vi "CFM_DAQ_SIMULACION.vi"() -> ()   [LabVIEW 2020]
panel:
  in  "stop":bool
  out "reinicio":bool
  out "M54":bool
  out "M53":bool
  out "M52":bool
  out "M51":bool
  in  "ACTUADOR RECHAZO":bool
  out "M50":bool
  out "M49":bool
  out "M48":bool
  out "M47":bool
  out "M46":bool
  out "M45":bool
  out "M44":bool
  out "TAPA NOPESO":bool
  out "M43":bool
  out "M42":bool
  out "M41":bool
  out "M40":bool
  out "M39":bool
  out "M38":bool
  out "M37":bool
  out "M36":bool
  out "M35":bool
  out "M34":bool
  out "TARRO NOPESO":bool
  out "DEPOSITO NOPESO":bool
  out "TAPA NOCOLOR":bool
  out "TARRO NOCOLOR":bool
  out "DEPOSITO NOCOLOR":bool
  out "CILINDRO RECHAZO1":bool
  out "VASTAGO RECHAZO":bool
  out "PINZA CERRADA":bool
  in  "PINZA ABIERTA":bool
  out "CILINDRO RECHAZO":bool
  out "ESTRUCTURA RECHAZO":bool
  out "M33":bool
  out "M32":bool
  out "M31":bool
  out "M30":bool
  out "M29":bool
  out "M28":bool
  out "M27":bool
  out "M26":bool
  out "TAPA AZUL":bool
  out "M25":bool
  out "M24":bool
  out "TAPA TARRO ROJO":bool
  in  "CILINDRO MODULO6":bool
  in  "VASTAGO MODULO6":bool
  in  "MODULO6":bool
  out "M23":bool
  out "M22":bool
  out "M21":bool
  out "ANALIZANDO\nCC":bool
  out "M20":bool
  out "balanza2":bool
  out "M19":bool
  out "M18":bool
  out "M17":bool
  out "M16":bool
  out "M15":bool
  out "M14":bool
  out "M13":bool
  out "M12":bool
  out "M11":bool
  out "M10":bool
  out "M9":bool
  out "M8":bool
  out "M7":bool
  out "M6":bool
  out "M5":bool
  out "M4":bool
  out "M3":bool
  out "M2":bool
  out "M1":bool
  out "tapa neutrop":bool
  out "cilindro3 tapado":bool
  out "vastago3 tapado":bool
  out "vastago4 tapado":bool
  out "cilindro2 tapado":bool
  in  "vastago2 tapado":bool
  out "cilindro1 tapado":bool
  in  "vastago1 tapado":bool
  out "estructura tapado":bool
  out "tarro llenop":bool
  out "tarro vaciop1":bool
  out "cilindros tolva":bool
  out "perta tolva1":bool
  out "puerta tolva2":bool
  out "dep inferior":bool
  out "dep superior":bool
  out "tolva vacia":bool
  out "cuadroblanco":bool
  out "vastagoaux1":bool
  out "tarro vaciop":bool
  out "estructura1":bool
  out "CILINDRO NUEVO":bool
  out "TAPA NEUTRO":bool
  out "BALANZA1":bool
  in  "BASTAGO TAPAS":bool
  out "PUERTA TOLVA":bool
  out "CAJA LLENA":bool
  out "TARRO VACIO":bool
  in  "BPESO NO":bool
  in  "BPESO SI":bool
  in  "BNO COLOR":bool
  in  "BROJO":bool
  in  "BAZUL":bool
  in  "REINICIAR\nCONTEO":bool
  out "FINALIZADOS\nRECHAZADOS":dbl
  out "FINALIZADOS\nROJOS":dbl
  out "FINALIZADOS\nAZULES":dbl
  out "AZUL":bool
  out "ROJO":bool
  out "NO \nCOLOR":bool
  out "PESO\nNO":bool
  out "PESO\nSI":bool
  in  "RESET":bool
  in  "INICIO":bool
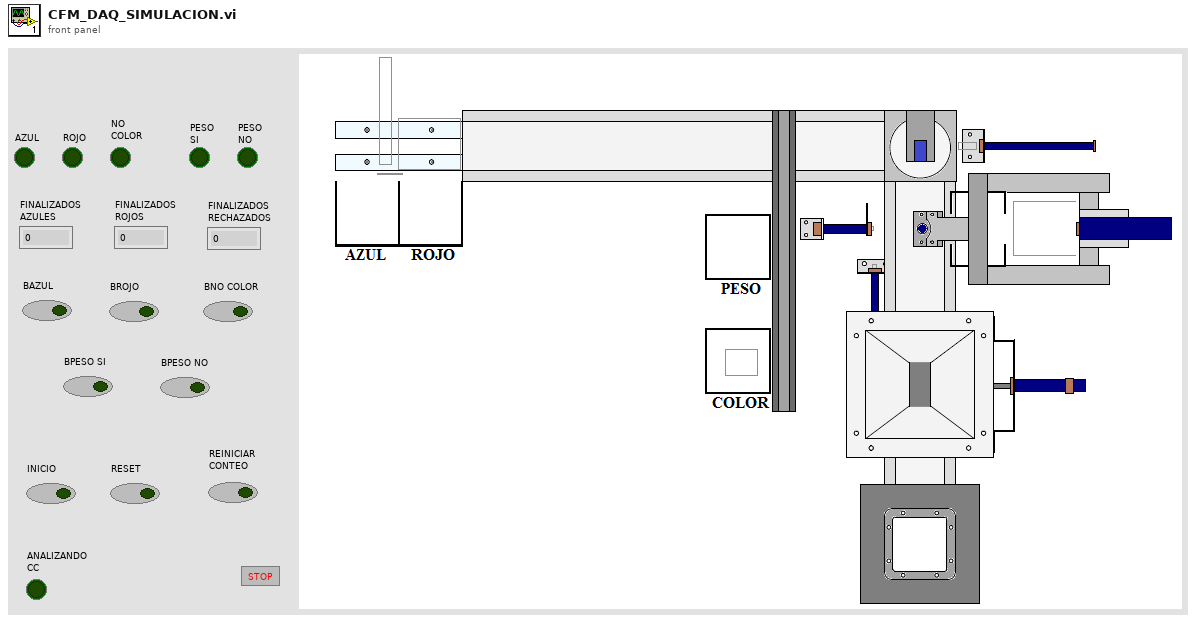
[diagram p1: front panel]
diagram:
  n1 = while {
    stop <- "stop" stop-if-true
    n2 = property on="M53" class="Bool (strict)"("Visible"=FALSE) -> ()  [unwired: 2 in, 2 out]
    n3 = property on="M54" class="Bool (strict)"("Visible"=FALSE) -> ()  [unwired: 2 in, 2 out]
    n4 = property on="M52" class="Bool (strict)"("Visible"=FALSE) -> ()  [unwired: 2 in, 2 out]
    n5 = property on="M48" class="Bool (strict)"("Visible"=FALSE) -> ()  [unwired: 2 in, 2 out]
    n6 = property on="M43" class="Bool (strict)"("Visible"=FALSE) -> ()  [unwired: 2 in, 2 out]
    n7 = property on="M47" class="Bool (strict)"("Visible"=FALSE) -> ()  [unwired: 2 in, 2 out]
    n8 = property on="M42" class="Bool (strict)"("Visible"=FALSE) -> ()  [unwired: 2 in, 2 out]
    n9 = property on="M41" class="Bool (strict)"("Visible"=FALSE) -> ()  [unwired: 2 in, 2 out]
    n10 = property on="M49" class="Bool (strict)"("Visible"=FALSE) -> ()  [unwired: 2 in, 2 out]
    n11 = property on="M40" class="Bool (strict)"("Visible"=FALSE) -> ()  [unwired: 2 in, 2 out]
    n12 = property on="M45" class="Bool (strict)"("Visible"=FALSE) -> ()  [unwired: 2 in, 2 out]
    n13 = property on="M46" class="Bool (strict)"("Visible"=FALSE) -> ()  [unwired: 2 in, 2 out]
    n14 = property on="reinicio" class="Bool (strict)"("Visible"=FALSE) -> ()  [unwired: 2 in, 2 out]
    n15 = property on="M24" class="Bool (strict)"("Visible"=FALSE) -> ()  [unwired: 2 in, 2 out]
    n16 = property on="M39" class="Bool (strict)"("Visible"=FALSE) -> ()  [unwired: 2 in, 2 out]
    n17 = property on="M44" class="Bool (strict)"("Visible"=FALSE) -> ()  [unwired: 2 in, 2 out]
    n18 = property on="M50" class="Bool (strict)"("Visible"=FALSE) -> ()  [unwired: 2 in, 2 out]
    n19 = property on="M25" class="Bool (strict)"("Visible"=FALSE) -> ()  [unwired: 2 in, 2 out]
    n20 = property on="M37" class="Bool (strict)"("Visible"=FALSE) -> ()  [unwired: 2 in, 2 out]
    n21 = property on="M38" class="Bool (strict)"("Visible"=FALSE) -> ()  [unwired: 2 in, 2 out]
    n22 = property on="M23" class="Bool (strict)"("Visible"=FALSE) -> ()  [unwired: 2 in, 2 out]
    n23 = property on="M22" class="Bool (strict)"("Visible"=FALSE) -> ()  [unwired: 2 in, 2 out]
    n24 = property on="M51" class="Bool (strict)"("Visible"=FALSE) -> ()  [unwired: 2 in, 2 out]
    n25 = property on="M36" class="Bool (strict)"("Visible"=FALSE) -> ()  [unwired: 2 in, 2 out]
    n26 = property on="M21" class="Bool (strict)"("Visible"=FALSE) -> ()  [unwired: 2 in, 2 out]
    n27 = property on="M27" class="Bool (strict)"("Visible"=FALSE) -> ()  [unwired: 2 in, 2 out]
    n28 = property on="M33" class="Bool (strict)"("Visible"=FALSE) -> ()  [unwired: 2 in, 2 out]
    n29 = property on="M2" class="Bool (strict)"("Visible"=FALSE) -> ()  [unwired: 2 in, 2 out]
    n30 = property on="M26" class="Bool (strict)"("Visible"=FALSE) -> ()  [unwired: 2 in, 2 out]
    n31 = property on="M35" class="Bool (strict)"("Visible"=FALSE) -> ()  [unwired: 2 in, 2 out]
    n32 = property on="M1" class="Bool (strict)"("Visible"=FALSE) -> ()  [unwired: 2 in, 2 out]
    n33 = property on="M32" class="Bool (strict)"("Visible"=FALSE) -> ()  [unwired: 2 in, 2 out]
    n34 = property on="M34" class="Bool (strict)"("Visible"=FALSE) -> ()  [unwired: 2 in, 2 out]
    n35 = property on="M13" class="Bool (strict)"("Visible"=FALSE) -> ()  [unwired: 2 in, 2 out]
    n36 = property on="M20" class="Bool (strict)"("Visible"=FALSE) -> ()  [unwired: 2 in, 2 out]
    n37 = property on="M29" class="Bool (strict)"("Visible"=FALSE) -> ()  [unwired: 2 in, 2 out]
    n38 = property on="M15" class="Bool (strict)"("Visible"=FALSE) -> ()  [unwired: 2 in, 2 out]
    n39 = property on="M28" class="Bool (strict)"("Visible"=FALSE) -> ()  [unwired: 2 in, 2 out]
    n40 = property on="M5" class="Bool (strict)"("Visible"=FALSE) -> ()  [unwired: 2 in, 2 out]
    n41 = property on="M3" class="Bool (strict)"("Visible"=FALSE) -> ()  [unwired: 2 in, 2 out]
    n42 = property on="M18" class="Bool (strict)"("Visible"=FALSE) -> ()  [unwired: 2 in, 2 out]
    n43 = property on="M19" class="Bool (strict)"("Visible"=FALSE) -> ()  [unwired: 2 in, 2 out]
    n44 = property on="M8" class="Bool (strict)"("Visible"=FALSE) -> ()  [unwired: 2 in, 2 out]
    n45 = property on="M7" class="Bool (strict)"("Visible"=FALSE) -> ()  [unwired: 2 in, 2 out]
    n46 = property on="M30" class="Bool (strict)"("Visible"=FALSE) -> ()  [unwired: 2 in, 2 out]
    n47 = property on="M6" class="Bool (strict)"("Visible"=FALSE) -> ()  [unwired: 2 in, 2 out]
    n48 = property on="M9" class="Bool (strict)"("Visible"=FALSE) -> ()  [unwired: 2 in, 2 out]
    n49 = property on="M17" class="Bool (strict)"("Visible"=FALSE) -> ()  [unwired: 2 in, 2 out]
    n50 = property on="M4" class="Bool (strict)"("Visible"=FALSE) -> ()  [unwired: 2 in, 2 out]
    n51 = property on="M10" class="Bool (strict)"("Visible"=FALSE) -> ()  [unwired: 2 in, 2 out]
    n52 = property on="M11" class="Bool (strict)"("Visible"=FALSE) -> ()  [unwired: 2 in, 2 out]
    n53 = property on="M14" class="Bool (strict)"("Visible"=FALSE) -> ()  [unwired: 2 in, 2 out]
    n54 = property on="M16" class="Bool (strict)"("Visible"=FALSE) -> ()  [unwired: 2 in, 2 out]
    n55 = property on="M12" class="Bool (strict)"("Visible"=FALSE) -> ()  [unwired: 2 in, 2 out]
    n56 = property on="M31" class="Bool (strict)"("Visible"=FALSE) -> ()  [unwired: 2 in, 2 out]
    n57 = property on="ACTUADOR RECHAZO" class="Bool (strict)"() -> ("Top"=w82:i32)  [unwired: 2 in, 2 out]
    n58 = property on="ACTUADOR RECHAZO" class="Bool (strict)"() -> ("Top"=w67:i32)  [unwired: 2 in, 2 out]
    n59 = property on="ACTUADOR RECHAZO" class="Bool (strict)"() -> ("Top"=w97:i32)  [unwired: 2 in, 2 out]
    n60 = property on="ACTUADOR RECHAZO" class="Bool (strict)"() -> ("Top"=w154:i32)  [unwired: 2 in, 2 out]
    n61 = local read "BNO COLOR"() -> (w121:bool)
    n62 = property on="ACTUADOR RECHAZO" class="Bool (strict)"() -> ("Top"=w139:i32)  [unwired: 2 in, 2 out]
    n63 = property on="VASTAGO MODULO6" class="Bool (strict)"() -> ("Top"=w232:i32)  [unwired: 2 in, 2 out]
    n64 = property on="VASTAGO MODULO6" class="Bool (strict)"() -> ("Top"=w195:i32)  [unwired: 2 in, 2 out]
    n65 = property on="VASTAGO MODULO6" class="Bool (strict)"() -> ("Top"=w190:i32)  [unwired: 2 in, 2 out]
    n66 = property on="VASTAGO MODULO6" class="Bool (strict)"() -> ("Top"=w237:i32)  [unwired: 2 in, 2 out]
    n67 = local read "BPESO NO"() -> (w122:bool)
    n68 = property on="TAPA TARRO ROJO" class="Bool (strict)"() -> ("Left"=w242:i32)  [unwired: 2 in, 2 out]
    n69 = local read "BPESO NO"() -> (w168:bool)
    n70 = property on="PINZA CERRADA" class="Bool (strict)"() -> ("Top"=w77:i32)  [unwired: 2 in, 2 out]
    n71 = property on="PINZA CERRADA" class="Bool (strict)"() -> ("Top"=w129:i32)  [unwired: 2 in, 2 out]
    n72 = property on="PINZA CERRADA" class="Bool (strict)"() -> ("Top"=w87:i32)  [unwired: 2 in, 2 out]
    n73 = property on="PINZA CERRADA" class="Bool (strict)"() -> ("Top"=w72:i32)  [unwired: 2 in, 2 out]
    n74 = property on="vastago4 tapado" class="Bool (strict)"() -> ("Top"=w300:i32)  [unwired: 2 in, 2 out]
    n75 = property on="TAPA NOCOLOR" class="Bool (strict)"() -> ("Left"=w159:i32)  [unwired: 2 in, 2 out]
    n76 = property on="BASTAGO TAPAS" class="Bool (strict)"() -> ("Left"=w305:i32)  [unwired: 2 in, 2 out]
    n77 = property on="PINZA CERRADA" class="Bool (strict)"() -> ("Top"=w149:i32)  [unwired: 2 in, 2 out]
    n78 = property on="PINZA CERRADA" class="Bool (strict)"() -> ("Top"=w144:i32)  [unwired: 2 in, 2 out]
    n79 = property on="vastago4 tapado" class="Bool (strict)"() -> ("Top"=w295:i32)  [unwired: 2 in, 2 out]
    n80 = property on="CILINDRO NUEVO" class="Bool (strict)"() -> ("Left"=w290:i32)  [unwired: 2 in, 2 out]
    n81 = property on="PINZA CERRADA" class="Bool (strict)"() -> ("Top"=w92:i32)  [unwired: 2 in, 2 out]
    n82 = property on="vastago3 tapado" class="Bool (strict)"() -> ("Top"=w280:i32)  [unwired: 2 in, 2 out]
    n83 = local read "BNO COLOR"() -> (w169:bool)
    n84 = property on="PINZA CERRADA" class="Bool (strict)"() -> ("Top"=w134:i32)  [unwired: 2 in, 2 out]
    n85 = property on="TAPA NOPESO" class="Bool (strict)"() -> ("Left"=w102:i32)  [unwired: 2 in, 2 out]
    n86 = property on="balanza2" class="Bool (strict)"() -> ("Left"=w109:i32)  [unwired: 2 in, 2 out]
    n87 = property on="TAPA NEUTRO" class="Bool (strict)"() -> ("Top"=w275:i32)  [unwired: 2 in, 2 out]
    n88 = property on="TAPA NEUTRO" class="Bool (strict)"() -> ("Top"=w265:i32)  [unwired: 2 in, 2 out]
    n89 = property on="PUERTA TOLVA" class="Bool (strict)"() -> ("Left"=w330:i32)  [unwired: 2 in, 2 out]
    n90 = property on="PUERTA TOLVA" class="Bool (strict)"() -> ("Left"=w325:i32)  [unwired: 2 in, 2 out]
    n91 = property on="tapa neutrop" class="Bool (strict)"() -> ("Top"=w285:i32)  [unwired: 2 in, 2 out]
    n92 = property on="TARRO VACIO" class="Bool (strict)"() -> ("Top"=w335:i32)  [unwired: 2 in, 2 out]
    n93 = property on="vastagoaux1" class="Bool (strict)"() -> ("Top"=w345:i32)  [unwired: 2 in, 2 out]
    n94 = local read "BPESO SI"() -> (w224:bool)
    n95 = property on="balanza2" class="Bool (strict)"() -> ("Left"=w119:i32)  [unwired: 2 in, 2 out]
    n96 = local read "BPESO SI"() -> (w230:bool)
    n97 = property on="puerta tolva2" class="Bool (strict)"() -> ("Left"=w320:i32)  [unwired: 2 in, 2 out]
    n98 = property on="puerta tolva2" class="Bool (strict)"() -> ("Left"=w315:i32)  [unwired: 2 in, 2 out]
    n99 = local read "BPESO NO"() -> (w124:bool)
    n100 = property on="vastagoaux1" class="Bool (strict)"() -> ("Top"=w350:i32)  [unwired: 2 in, 2 out]
    n101 = property on="vastagoaux1" class="Bool (strict)"() -> ("Top"=w340:i32)  [unwired: 2 in, 2 out]
    n102 = property on="TAPA AZUL" class="Bool (strict)"() -> ("Left"=w205:i32)  [unwired: 2 in, 2 out]
    n103 = property on="MODULO6" class="Bool (strict)"() -> ("Left"=w200:i32)  [unwired: 2 in, 2 out]
    n104 = property on="MODULO6" class="Bool (strict)"() -> ("Left"=w185:i32)  [unwired: 2 in, 2 out]
    n105 = property on="CAJA LLENA" class="Bool (strict)"() -> ("Top"=w310:i32)  [unwired: 2 in, 2 out]
    n106 = property on="BALANZA1" class="Bool (strict)"() -> ("Top"=w270:i32)  [unwired: 2 in, 2 out]
    n107 = property on="balanza2" class="Bool (strict)"() -> ("Left"=w114:i32)  [unwired: 2 in, 2 out]
    n108 = property on="balanza2" class="Bool (strict)"() -> ("Left"=w220:i32)  [unwired: 2 in, 2 out]
    n109 = local read "BROJO"() -> (w229:bool)
    n110 = local read "BAZUL"() -> (w225:bool)
    n111 = property on="balanza2" class="Bool (strict)"() -> ("Left"=w259:i32)  [unwired: 2 in, 2 out]
    n112 = property on="balanza2" class="Bool (strict)"() -> ("Left"=w164:i32)  [unwired: 2 in, 2 out]
    n113 = property on="balanza2" class="Bool (strict)"() -> ("Left"=w210:i32)  [unwired: 2 in, 2 out]
    n114 = property on="balanza2" class="Bool (strict)"() -> ("Left"=w176:i32)  [unwired: 2 in, 2 out]
    n115 = property on="balanza2" class="Bool (strict)"() -> ("Left"=w247:i32)  [unwired: 2 in, 2 out]
    n116 = property on="balanza2" class="Bool (strict)"() -> ("Left"=w215:i32)  [unwired: 2 in, 2 out]
    n117 = property on="balanza2" class="Bool (strict)"() -> ("Left"=w171:i32)  [unwired: 2 in, 2 out]
    n118 = property on="balanza2" class="Bool (strict)"() -> ("Left"=w252:i32)  [unwired: 2 in, 2 out]
    n119 = local read "reinicio"() -> (w63:bool)
    n120 = local read "INICIO"() -> (w64:bool)
    n121 = Not(x=w168) -> (.not. x?=w180:bool)
    n122 = local read "M46"() -> (w106:bool)
    n123 = And(x=w122, y=w121) -> (x .and. y?=w123:bool)
    n124 = Less?(x=w119, y=965) -> (x < y?=w120:bool)
    n125 = local read "M52"() -> (w79:bool)
    n126 = local read "M47"() -> (w104:bool)
    n127 = local read "M45"() -> (w111:bool)
    n128 = local read "M43"() -> (w131:bool)
    n129 = local read "M50"() -> (w89:bool)
    n130 = local read "M44"() -> (w116:bool)
    n131 = Greater?(x=w109, y=977) -> (0:w110:bool)
    n132 = local read "M51"() -> (w84:bool)
    n133 = local read "M54"() -> (w69:bool)
    n134 = local read "M19"() -> (w262:bool)
    n135 = local read "M25"() -> (w234:bool)
    n136 = local read "M26"() -> (w222:bool)
    n137 = local read "M36"() -> (w166:bool)
    n138 = local read "M37"() -> (w161:bool)
    n139 = local read "M53"() -> (w74:bool)
    n140 = local read "M28"() -> (w212:bool)
    n141 = local read "M48"() -> (w99:bool)
    n142 = local read "M10"() -> (w307:bool)
    n143 = local read "M14"() -> (w287:bool)
    n144 = local read "M16"() -> (w277:bool)
    n145 = local read "M20"() -> (w257:bool)
    n146 = local read "M30"() -> (w202:bool)
    n147 = local read "M31"() -> (w197:bool)
    n148 = local read "M33"() -> (w187:bool)
    n149 = local read "M39"() -> (w151:bool)
    n150 = local read "M40"() -> (w146:bool)
    n151 = local read "M23"() -> (w244:bool)
    n152 = local read "M29"() -> (w207:bool)
    n153 = local read "M34"() -> (w178:bool)
    n154 = local read "M41"() -> (w141:bool)
    n155 = local read "M12"() -> (w297:bool)
    n156 = local read "M19"() -> (w227:bool)
    n157 = local read "M32"() -> (w192:bool)
    n158 = local read "M19"() -> (w182:bool)
    n159 = local read "M38"() -> (w156:bool)
    n160 = local read "M49"() -> (w94:bool)
    n161 = local read "M11"() -> (w302:bool)
    n162 = local read "M17"() -> (w272:bool)
    n163 = local read "M18"() -> (w267:bool)
    n164 = local read "M22"() -> (w249:bool)
    n165 = local read "M24"() -> (w239:bool)
    n166 = local read "M27"() -> (w217:bool)
    n167 = local read "M35"() -> (w173:bool)
    n168 = local read "M42"() -> (w136:bool)
    n169 = local read "M19"() -> (w126:bool)
    n170 = local read "M2"() -> (w347:bool)
    n171 = local read "M15"() -> (w282:bool)
    n172 = local read "M1"() -> (w352:bool)
    n173 = local read "M21"() -> (w254:bool)
    n174 = local read "M4"() -> (w337:bool)
    n175 = local read "M13"() -> (w292:bool)
    n176 = local read "M6"() -> (w327:bool)
    n177 = local read "M8"() -> (w317:bool)
    n178 = Less?(x=w114, y=900) -> (x < y?=w115:bool)
    n179 = local read "M3"() -> (w342:bool)
    n180 = local read "M5"() -> (w332:bool)
    n181 = local read "M9"() -> (w312:bool)
    n182 = local read "M7"() -> (w322:bool)
    n183 = Equal?(x=420, y=w350) -> (x = y?=w351:bool)
    n184 = Less?(x=w102, y=737) -> (x < y?=w103:bool)
    n185 = property on="BAZUL" class="Bool (strict)"("Visible"=TRUE) -> ()  [unwired: 2 in, 2 out]
    n186 = Greater?(x=w195, y=55) -> (0:w196:bool)
    n187 = Less?(x=w129, y=317) -> (x < y?=w130:bool)
    n188 = Greater?(x=w77, y=396) -> (0:w78:bool)
    n189 = And(x=w229, y=w230) -> (x .and. y?=w261:bool)
    n190 = Less?(x=w275, y=67) -> (x < y?=w276:bool)
    n191 = And(x=w225, y=w224) -> (x .and. y?=w226:bool)
    n192 = Less?(x=w205, y=426) -> (x < y?=w206:bool)
    n193 = Greater?(x=w139, y=219) -> (0:w140:bool)
    n194 = Less?(x=w97, y=6) -> (x < y?=w98:bool)
    n195 = Less?(x=w87, y=317) -> (x < y?=w88:bool)
    n196 = property on="BROJO" class="Bool (strict)"("Visible"=TRUE) -> ()  [unwired: 2 in, 2 out]
    n197 = Less?(x=w232, y=-10) -> (x < y?=w233:bool)
    n198 = Less?(x=w159, y=737) -> (x < y?=w160:bool)
    n199 = Greater?(x=w67, y=219) -> (0:w68:bool)
    n200 = Less?(x=w305, y=911) -> (x < y?=w306:bool)
    n201 = Greater?(x=w285, y=367) -> (0:w286:bool)
    n202 = Less?(x=w215, y=900) -> (x < y?=w216:bool)
    n203 = Greater?(x=w210, y=977) -> (0:w211:bool)
    n204 = Greater?(x=w185, y=377) -> (0:w186:bool)
    n205 = Less?(x=w144, y=317) -> (x < y?=w145:bool)
    n206 = Greater?(x=w92, y=396) -> (0:w93:bool)
    n207 = Greater?(x=w340, y=383) -> (0:w341:bool)
    n208 = Less?(x=w335, y=252) -> (x < y?=w336:bool)
    n209 = Greater?(x=w300, y=258) -> (0:w301:bool)
    n210 = Less?(x=w259, y=965) -> (x < y?=w256:bool)
    n211 = Greater?(x=w237, y=38) -> (0:w238:bool)
    n212 = And(x=w169, y=w180) -> (x .and. y?=w181:bool)
    n213 = Less?(x=w72, y=317) -> (x < y?=w73:bool)
    n214 = Less?(x=w242, y=426) -> (x < y?=w243:bool)
    n215 = Less?(x=w220, y=965) -> (x < y?=w221:bool)
    n216 = Less?(x=w200, y=316) -> (x < y?=w201:bool)
    n217 = Less?(x=w190, y=10) -> (x < y?=w191:bool)
    n218 = Less?(x=w176, y=965) -> (x < y?=w177:bool)
    n219 = Less?(x=w171, y=900) -> (x < y?=w172:bool)
    n220 = Greater?(x=w164, y=977) -> (0:w165:bool)
    n221 = Less?(x=w154, y=6) -> (x < y?=w155:bool)
    n222 = Greater?(x=w134, y=396) -> (0:w135:bool)
    n223 = Or(x=w124, y=w123) -> (x .or. y?=w125:bool)
    n224 = Less?(x=w325, y=931) -> (x < y?=w326:bool)
    n225 = Less?(x=w295, y=227) -> (x < y?=w296:bool)
    n226 = Less?(x=w270, y=109) -> (x < y?=w271:bool)
    n227 = Greater?(x=w247, y=977) -> (0:w248:bool)
    n228 = Greater?(x=w149, y=396) -> (0:w150:bool)
    n229 = Greater?(x=w82, y=100) -> (0:w83:bool)
    n230 = Less?(x=w345, y=386) -> (x < y?=w346:bool)
    n231 = Less?(x=w320, y=425) -> (x < y?=w321:bool)
    n232 = Less?(x=w310, y=97) -> (x < y?=w311:bool)
    n233 = Less?(x=w265, y=16) -> (x < y?=w266:bool)
    n234 = Greater?(x=w315, y=449) -> (0:w316:bool)
    n235 = Less?(x=w290, y=870) -> (x < y?=w291:bool)
    n236 = Greater?(x=w330, y=950) -> (0:w331:bool)
    n237 = Less?(x=w280, y=207) -> (x < y?=w281:bool)
    n238 = Less?(x=w252, y=900) -> (x < y?=w253:bool)
    n239 = local read "RESET"() -> (w62:bool)
    n240 = Or(x=w64, y=w63) -> (x .or. y?=w65:bool)
    n241 = And(x=w277, y=w276) -> (x .and. y?=w278:bool)
    n242 = And(x=w161, y=w160) -> (x .and. y?=w162:bool)
    n243 = And(x=w352, y=w351) -> (x .and. y?=w353:bool)
    n244 = And(x=w287, y=w286) -> (x .and. y?=w288:bool)
    n245 = And(x=w234, y=w233) -> (x .and. y?=w235:bool)
    n246 = And(x=w146, y=w145) -> (x .and. y?=w147:bool)
    n247 = And(x=w131, y=w130) -> (x .and. y?=w132:bool)
    n248 = And(x=w111, y=w115) -> (x .and. y?=w112:bool)
    n249 = And(x=w106, y=w110) -> (x .and. y?=w107:bool)
    n250 = And(x=w79, y=w78) -> (x .and. y?=w80:bool)
    n251 = And(x=w337, y=w336) -> (x .and. y?=w338:bool)
    n252 = And(x=w227, y=w226) -> (x .and. y?=w228:bool)
    n253 = And(x=w222, y=w221) -> (x .and. y?=w223:bool)
    n254 = And(x=w178, y=w177) -> (x .and. y?=w179:bool)
    n255 = And(x=w166, y=w165) -> (x .and. y?=w167:bool)
    n256 = And(x=w116, y=w120) -> (x .and. y?=w117:bool)
    n257 = And(x=w347, y=w346) -> (x .and. y?=w348:bool)
    n258 = And(x=w327, y=w326) -> (x .and. y?=w328:bool)
    n259 = And(x=w272, y=w271) -> (x .and. y?=w273:bool)
    n260 = And(x=w244, y=w243) -> (x .and. y?=w245:bool)
    n261 = And(x=w192, y=w191) -> (x .and. y?=w193:bool)
    n262 = And(x=w151, y=w150) -> (x .and. y?=w152:bool)
    n263 = And(x=w104, y=w103) -> (x .and. y?=w105:bool)
    n264 = And(x=w307, y=w306) -> (x .and. y?=w308:bool)
    n265 = And(x=w302, y=w301) -> (x .and. y?=w303:bool)
    n266 = And(x=w297, y=w296) -> (x .and. y?=w298:bool)
    n267 = And(x=w267, y=w266) -> (x .and. y?=w268:bool)
    n268 = And(x=w262, y=w261) -> (x .and. y?=w263:bool)
    n269 = And(x=w257, y=w256) -> (x .and. y?=w260:bool)
    n270 = And(x=w249, y=w248) -> (x .and. y?=w250:bool)
    n271 = And(x=w239, y=w238) -> (x .and. y?=w240:bool)
    n272 = And(x=w212, y=w211) -> (x .and. y?=w213:bool)
    n273 = And(x=w207, y=w206) -> (x .and. y?=w208:bool)
    n274 = And(x=w202, y=w201) -> (x .and. y?=w203:bool)
    n275 = And(x=w182, y=w181) -> (x .and. y?=w183:bool)
    n276 = And(x=w173, y=w172) -> (x .and. y?=w174:bool)
    n277 = And(x=w141, y=w140) -> (x .and. y?=w142:bool)
    n278 = And(x=w99, y=w98) -> (x .and. y?=w100:bool)
    n279 = And(x=w89, y=w88) -> (x .and. y?=w90:bool)
    n280 = And(x=w74, y=w73) -> (x .and. y?=w75:bool)
    n281 = And(x=w69, y=w68) -> (x .and. y?=w70:bool)
    n282 = And(x=w342, y=w341) -> (x .and. y?=w343:bool)
    n283 = And(x=w332, y=w331) -> (x .and. y?=w333:bool)
    n284 = And(x=w317, y=w316) -> (x .and. y?=w318:bool)
    n285 = And(x=w312, y=w311) -> (x .and. y?=w313:bool)
    n286 = And(x=w217, y=w216) -> (x .and. y?=w218:bool)
    n287 = And(x=w197, y=w196) -> (x .and. y?=w198:bool)
    n288 = And(x=w187, y=w186) -> (x .and. y?=w188:bool)
    n289 = And(x=w156, y=w155) -> (x .and. y?=w157:bool)
    n290 = And(x=w136, y=w135) -> (x .and. y?=w137:bool)
    n291 = And(x=w322, y=w321) -> (x .and. y?=w323:bool)
    n292 = And(x=w292, y=w291) -> (x .and. y?=w293:bool)
    n293 = And(x=w254, y=w253) -> (x .and. y?=w255:bool)
    n294 = And(x=w84, y=w83) -> (x .and. y?=w85:bool)
    n295 = And(x=w282, y=w281) -> (x .and. y?=w283:bool)
    n296 = And(x=w94, y=w93) -> (x .and. y?=w95:bool)
    n297 = And(x=w126, y=w125) -> (x .and. y?=w127:bool)
    n298 = case shown="True" w198 {
      frame False {
      }
      frame True {
        n299 = local read "FINALIZADOS\nAZULES"() -> (w855:dbl)
        n300 = Increment(x=w855) -> (x+1=w854:dbl)
        n301 = local write "FINALIZADOS\nAZULES"(w854) -> ()
        n302 = while {
          stop <- w856 stop-if-true
          n303 = property on="VASTAGO MODULO6" class="Bool (strict)"() -> ("Top"=w864:i32)  [unwired: 2 in, 2 out]
          n304 = Subtract(x=w864, y=2) -> (x-y=w862:i32)
          n305 = property on="VASTAGO MODULO6" class="Bool (strict)"("Top"=w862) -> ()  [unwired: 2 in, 2 out]
          n306 = Wait (ms)(milliseconds to wait=u32 0) -> ()  [unwired: 1 out]
          n307 = local read "RESET"() -> (w857:bool)
          n308 = property on="VASTAGO MODULO6" class="Bool (strict)"() -> ("Top"=w860:i32)  [unwired: 2 in, 2 out]
          n309 = Less?(x=w860, y=-10) -> (x < y?=w858:bool)
          n310 = Or(x=w858, y=w857) -> (x .or. y?=w856:bool)
        }
        n311 = local write "AZUL"(FALSE ("AZUL")) -> ()
        n312 = local write "PESO\nSI"(FALSE ("PESO\nSI")) -> ()
        n313 = local write "M31"(FALSE ("M31")) -> ()
        n314 = local write "M32"(TRUE ("M32")) -> ()
      }
    }
    n315 = case shown="True" w65 {
      frame False {
      }
      frame True {
        n316 = property on="TARRO VACIO" class="Bool (strict)"("Visible"=TRUE) -> ()  [unwired: 2 in, 2 out]
        n317 = property on="TAPA NEUTRO" class="Bool (strict)"("Visible"=TRUE) -> ()  [unwired: 2 in, 2 out]
        n318 = property on="estructura1" class="Bool (strict)"("Visible"=TRUE) -> ()  [unwired: 2 in, 2 out]
        n319 = property on="tarro vaciop" class="Bool (strict)"("Visible"=TRUE) -> ()  [unwired: 2 in, 2 out]
        n320 = property on="vastagoaux1" class="Bool (strict)"("Visible"=TRUE) -> ()  [unwired: 2 in, 2 out]
        n321 = property on="cuadroblanco" class="Bool (strict)"("Visible"=TRUE) -> ()  [unwired: 2 in, 2 out]
        n322 = property on="vastagoaux1" class="Bool (strict)"("Top"=420 ("Position:Top")) -> ()  [unwired: 2 in, 2 out]
        n323 = property on="TAPA NEUTRO" class="Bool (strict)"("Top"=96 ("Position:Top")) -> ()  [unwired: 2 in, 2 out]
        n324 = property on="TARRO VACIO" class="Bool (strict)"("Top"=412 ("Position:Top")) -> ()  [unwired: 2 in, 2 out]
        n325 = property on="PUERTA TOLVA" class="Bool (strict)"("Left"=929 ("Position:Left")) -> ()  [unwired: 2 in, 2 out]
        n326 = property on="CAJA LLENA" class="Bool (strict)"("Top"=250 ("Position:Top")) -> ()  [unwired: 2 in, 2 out]
        n327 = property on="BALANZA1" class="Bool (strict)"("Top"=146 ("Position:Top")) -> ()  [unwired: 2 in, 2 out]
        n328 = property on="CAJA LLENA" class="Bool (strict)"("Visible"=FALSE) -> ()  [unwired: 2 in, 2 out]
        n329 = property on="dep inferior" class="Bool (strict)"("Visible"=FALSE) -> ()  [unwired: 2 in, 2 out]
        n330 = property on="dep superior" class="Bool (strict)"("Visible"=FALSE) -> ()  [unwired: 2 in, 2 out]
        n331 = property on="cilindros tolva" class="Bool (strict)"("Visible"=FALSE) -> ()  [unwired: 2 in, 2 out]
        n332 = property on="puerta tolva2" class="Bool (strict)"("Visible"=FALSE) -> ()  [unwired: 2 in, 2 out]
        n333 = property on="perta tolva1" class="Bool (strict)"("Visible"=FALSE) -> ()  [unwired: 2 in, 2 out]
        n334 = local write "M1"(TRUE ("M1")) -> ()
        n335 = property on="CILINDRO NUEVO" class="Bool (strict)"("Left"=869 ("Position:Left")) -> ()  [unwired: 2 in, 2 out]
        n336 = property on="BASTAGO TAPAS" class="Bool (strict)"("Left"=973 ("Position:Left")) -> ()  [unwired: 2 in, 2 out]
        n337 = property on="TAPA NEUTRO" class="Bool (strict)"("Left"=980 ("Position:Left")) -> ()  [unwired: 2 in, 2 out]
        n338 = property on="tarro vaciop" class="Bool (strict)"("Top"=358 ("Position:Top")) -> ()  [unwired: 2 in, 2 out]
        n339 = property on="puerta tolva2" class="Bool (strict)"("Left"=450 ("Position:Left")) -> ()  [unwired: 2 in, 2 out]
        n340 = property on="perta tolva1" class="Bool (strict)"("Left"=450 ("Position:Left")) -> ()  [unwired: 2 in, 2 out]
        n341 = local write "reinicio"(FALSE ("reinicio")) -> ()
        n342 = property on="tolva vacia" class="Bool (strict)"("Visible"=FALSE) -> ()  [unwired: 2 in, 2 out]
        n343 = property on="tarro vaciop1" class="Bool (strict)"("Visible"=FALSE) -> ()  [unwired: 2 in, 2 out]
        n344 = property on="tarro llenop" class="Bool (strict)"("Visible"=FALSE) -> ()  [unwired: 2 in, 2 out]
        n345 = property on="estructura tapado" class="Bool (strict)"("Visible"=FALSE) -> ()  [unwired: 2 in, 2 out]
        n346 = property on="tapa neutrop" class="Bool (strict)"("Visible"=FALSE) -> ()  [unwired: 2 in, 2 out]
        n347 = property on="vastago1 tapado" class="Bool (strict)"("Visible"=FALSE) -> ()  [unwired: 2 in, 2 out]
        n348 = property on="tapa neutrop" class="Bool (strict)"("Left"=527 ("Position:Left")) -> ()  [unwired: 2 in, 2 out]
        n349 = property on="tapa neutrop" class="Bool (strict)"("Top"=345 ("Position:Top")) -> ()  [unwired: 2 in, 2 out]
        n350 = property on="vastago1 tapado" class="Bool (strict)"("Left"=361 ("Position:Left")) -> ()  [unwired: 2 in, 2 out]
        n351 = property on="vastago2 tapado" class="Bool (strict)"("Left"=626 ("Position:Left")) -> ()  [unwired: 2 in, 2 out]
        n352 = property on="vastago3 tapado" class="Bool (strict)"("Top"=206 ("Position:Top")) -> ()  [unwired: 2 in, 2 out]
        n353 = property on="vastago4 tapado" class="Bool (strict)"("Top"=226 ("Position:Top")) -> ()  [unwired: 2 in, 2 out]
        n354 = property on="cilindro1 tapado" class="Bool (strict)"("Visible"=FALSE) -> ()  [unwired: 2 in, 2 out]
        n355 = property on="vastago2 tapado" class="Bool (strict)"("Visible"=FALSE) -> ()  [unwired: 2 in, 2 out]
        n356 = property on="cilindro2 tapado" class="Bool (strict)"("Visible"=FALSE) -> ()  [unwired: 2 in, 2 out]
        n357 = property on="vastago3 tapado" class="Bool (strict)"("Visible"=FALSE) -> ()  [unwired: 2 in, 2 out]
        n358 = property on="cilindro3 tapado" class="Bool (strict)"("Visible"=FALSE) -> ()  [unwired: 2 in, 2 out]
        n359 = property on="vastago4 tapado" class="Bool (strict)"("Visible"=FALSE) -> ()  [unwired: 2 in, 2 out]
        n360 = property on="balanza2" class="Bool (strict)"("Left"=978 ("Position:Left")) -> ()  [unwired: 2 in, 2 out]
      }
    }
    n361 = case shown="True" w353 {
      frame False {
      }
      frame True {
        n362 = while {
          stop <- w1337 stop-if-true
          n363 = property on="vastagoaux1" class="Bool (strict)"() -> ("Top"=w1343:i32)  [unwired: 2 in, 2 out]
          n364 = Subtract(x=w1343, y=1) -> (x-y=w1344:i32)
          n365 = property on="vastagoaux1" class="Bool (strict)"("Top"=w1344) -> ()  [unwired: 2 in, 2 out]
          n366 = Wait (ms)(milliseconds to wait=u32 0) -> ()  [unwired: 1 out]
          n367 = property on="vastagoaux1" class="Bool (strict)"() -> ("Top"=w1341:i32)  [unwired: 2 in, 2 out]
          n368 = local read "RESET"() -> (w1338:bool)
          n369 = Less?(x=w1341, y=386) -> (x < y?=w1339:bool)
          n370 = Or(x=w1339, y=w1338) -> (x .or. y?=w1337:bool)
        }
        n371 = local write "M1"(FALSE ("M1")) -> ()
        n372 = local write "M2"(TRUE ("M2")) -> ()
      }
    }
    n373 = case shown="True" w348 {
      frame False {
      }
      frame True {
        n374 = while {
          stop <- w1322 stop-if-true
          n375 = property on="vastagoaux1" class="Bool (strict)"() -> ("Top"=w1333:i32)  [unwired: 2 in, 2 out]
          n376 = Add(x=w1333, y=1) -> (x+y=w1331:i32)
          n377 = property on="vastagoaux1" class="Bool (strict)"("Top"=w1331) -> ()  [unwired: 2 in, 2 out]
          n378 = property on="tarro vaciop" class="Bool (strict)"() -> ("Top"=w1330:i32)  [unwired: 2 in, 2 out]
          n379 = Add(x=w1330, y=1) -> (x+y=w1328:i32)
          n380 = property on="tarro vaciop" class="Bool (strict)"("Top"=w1328) -> ()  [unwired: 2 in, 2 out]
          n381 = Wait (ms)(milliseconds to wait=u32 0) -> ()  [unwired: 1 out]
          n382 = property on="vastagoaux1" class="Bool (strict)"() -> ("Top"=w1327:i32)  [unwired: 2 in, 2 out]
          n383 = local read "RESET"() -> (w1323:bool)
          n384 = Greater?(x=w1327, y=419) -> (0:w1324:bool)
          n385 = Or(x=w1324, y=w1323) -> (x .or. y?=w1322:bool)
        }
        n386 = local write "M2"(FALSE ("M2")) -> ()
        n387 = local write "M3"(TRUE ("M3")) -> ()
      }
    }
    n388 = case shown="True" w343 {
      frame False {
      }
      frame True {
        n389 = property on="estructura1" class="Bool (strict)"("Visible"=FALSE) -> ()  [unwired: 2 in, 2 out]
        n390 = property on="tarro vaciop" class="Bool (strict)"("Visible"=FALSE) -> ()  [unwired: 2 in, 2 out]
        n391 = property on="vastagoaux1" class="Bool (strict)"("Visible"=FALSE) -> ()  [unwired: 2 in, 2 out]
        n392 = property on="cuadroblanco" class="Bool (strict)"("Visible"=FALSE) -> ()  [unwired: 2 in, 2 out]
        n393 = while {
          stop <- w1312 stop-if-true
          n394 = property on="TARRO VACIO" class="Bool (strict)"() -> ("Top"=w1319:i32)  [unwired: 2 in, 2 out]
          n395 = Subtract(x=w1319, y=1) -> (x-y=w1317:i32)
          n396 = property on="TARRO VACIO" class="Bool (strict)"("Top"=w1317) -> ()  [unwired: 2 in, 2 out]
          n397 = Wait (ms)(milliseconds to wait=u32 0) -> ()  [unwired: 1 out]
          n398 = local read "RESET"() -> (w1313:bool)
          n399 = property on="TARRO VACIO" class="Bool (strict)"() -> ("Top"=w1316:i32)  [unwired: 2 in, 2 out]
          n400 = Less?(x=w1316, y=252) -> (x < y?=w1314:bool)
          n401 = Or(x=w1314, y=w1313) -> (x .or. y?=w1312:bool)
        }
        n402 = local write "M3"(FALSE ("M3")) -> ()
        n403 = local write "M4"(TRUE ("M4")) -> ()
      }
    }
    n404 = case shown="True" w333 {
      frame False {
      }
      frame True {
        n405 = property on="dep inferior" class="Bool (strict)"("Visible"=TRUE) -> ()  [unwired: 2 in, 2 out]
        n406 = property on="dep superior" class="Bool (strict)"("Visible"=FALSE) -> ()  [unwired: 2 in, 2 out]
        n407 = while {
          stop <- w1273 stop-if-true
          n408 = property on="PUERTA TOLVA" class="Bool (strict)"() -> ("Left"=w1284:i32)  [unwired: 2 in, 2 out]
          n409 = Subtract(x=w1284, y=1) -> (x-y=w1282:i32)
          n410 = property on="PUERTA TOLVA" class="Bool (strict)"("Left"=w1282) -> ()  [unwired: 2 in, 2 out]
          n411 = property on="perta tolva1" class="Bool (strict)"() -> ("Left"=w1278:i32)  [unwired: 2 in, 2 out]
          n412 = Add(x=w1278, y=1) -> (x+y=w1276:i32)
          n413 = property on="perta tolva1" class="Bool (strict)"("Left"=w1276) -> ()  [unwired: 2 in, 2 out]
          n414 = Wait (ms)(milliseconds to wait=u32 0) -> ()  [unwired: 1 out]
          n415 = local read "RESET"() -> (w1274:bool)
          n416 = property on="PUERTA TOLVA" class="Bool (strict)"() -> ("Left"=w1281:i32)  [unwired: 2 in, 2 out]
          n417 = Less?(x=w1281, y=930) -> (x < y?=w1279:bool)
          n418 = Or(x=w1279, y=w1274) -> (x .or. y?=w1273:bool)
        }
        n419 = local write "M5"(FALSE ("M5")) -> ()
        n420 = local write "M6"(TRUE ("M6")) -> ()
      }
    }
    n421 = case shown="True" w328 {
      frame False {
      }
      frame True {
        n422 = while {
          stop <- w1260 stop-if-true
          n423 = property on="puerta tolva2" class="Bool (strict)"() -> ("Left"=w1268:i32)  [unwired: 2 in, 2 out]
          n424 = Subtract(x=w1268, y=1) -> (x-y=w1266:i32)
          n425 = property on="puerta tolva2" class="Bool (strict)"("Left"=w1266) -> ()  [unwired: 2 in, 2 out]
          n426 = Wait (ms)(milliseconds to wait=u32 0) -> ()  [unwired: 1 out]
          n427 = local read "RESET"() -> (w1261:bool)
          n428 = property on="puerta tolva2" class="Bool (strict)"() -> ("Left"=w1265:i32)  [unwired: 2 in, 2 out]
          n429 = Less?(x=w1265, y=425) -> (x < y?=w1262:bool)
          n430 = Or(x=w1262, y=w1261) -> (x .or. y?=w1260:bool)
        }
        n431 = local write "M6"(FALSE ("M6")) -> ()
        n432 = local write "M7"(TRUE ("M7")) -> ()
      }
    }
    n433 = case shown="True" w323 {
      frame False {
      }
      frame True {
        n434 = property on="dep inferior" class="Bool (strict)"("Visible"=FALSE) -> ()  [unwired: 2 in, 2 out]
        n435 = property on="tarro llenop" class="Bool (strict)"("Visible"=TRUE) -> ()  [unwired: 2 in, 2 out]
        n436 = property on="tarro vaciop1" class="Bool (strict)"("Visible"=FALSE) -> ()  [unwired: 2 in, 2 out]
        n437 = while {
          stop <- w1249 stop-if-true
          n438 = property on="puerta tolva2" class="Bool (strict)"() -> ("Left"=w1257:i32)  [unwired: 2 in, 2 out]
          n439 = Add(x=w1257, y=1) -> (x+y=w1255:i32)
          n440 = property on="puerta tolva2" class="Bool (strict)"("Left"=w1255) -> ()  [unwired: 2 in, 2 out]
          n441 = Wait (ms)(milliseconds to wait=u32 0) -> ()  [unwired: 1 out]
          n442 = local read "RESET"() -> (w1250:bool)
          n443 = property on="puerta tolva2" class="Bool (strict)"() -> ("Left"=w1254:i32)  [unwired: 2 in, 2 out]
          n444 = Greater?(x=w1254, y=449) -> (0:w1251:bool)
          n445 = Or(x=w1251, y=w1250) -> (x .or. y?=w1249:bool)
        }
        n446 = local write "M7"(FALSE ("M7")) -> ()
        n447 = local write "M8"(TRUE ("M8")) -> ()
      }
    }
    n448 = case shown="True" w308 {
      frame False {
      }
      frame True {
        n449 = while {
          stop <- w1179 stop-if-true
          n450 = property on="vastago4 tapado" class="Bool (strict)"() -> ("Top"=w1187:i32)  [unwired: 2 in, 2 out]
          n451 = Add(x=w1187, y=1) -> (x+y=w1185:i32)
          n452 = property on="vastago4 tapado" class="Bool (strict)"("Top"=w1185) -> ()  [unwired: 2 in, 2 out]
          n453 = Wait (ms)(milliseconds to wait=u32 0) -> ()  [unwired: 1 out]
          n454 = local read "RESET"() -> (w1180:bool)
          n455 = property on="vastago4 tapado" class="Bool (strict)"() -> ("Top"=w1184:i32)  [unwired: 2 in, 2 out]
          n456 = Greater?(x=w1184, y=258) -> (0:w1181:bool)
          n457 = Or(x=w1181, y=w1180) -> (x .or. y?=w1179:bool)
        }
        n458 = local write "M10"(FALSE ("M10")) -> ()
        n459 = local write "M11"(TRUE ("M11")) -> ()
      }
    }
    n460 = case shown="True" w303 {
      frame False {
      }
      frame True {
        n461 = while {
          stop <- w1165 stop-if-true
          n462 = property on="tapa neutrop" class="Bool (strict)"() -> ("Top"=w1176:i32)  [unwired: 2 in, 2 out]
          n463 = Subtract(x=w1176, y=1) -> (x-y=w1174:i32)
          n464 = property on="tapa neutrop" class="Bool (strict)"("Top"=w1174) -> ()  [unwired: 2 in, 2 out]
          n465 = property on="vastago4 tapado" class="Bool (strict)"() -> ("Top"=w1173:i32)  [unwired: 2 in, 2 out]
          n466 = Subtract(x=w1173, y=1) -> (x-y=w1171:i32)
          n467 = property on="vastago4 tapado" class="Bool (strict)"("Top"=w1171) -> ()  [unwired: 2 in, 2 out]
          n468 = Wait (ms)(milliseconds to wait=u32 0) -> ()  [unwired: 1 out]
          n469 = local read "RESET"() -> (w1166:bool)
          n470 = property on="vastago4 tapado" class="Bool (strict)"() -> ("Top"=w1170:i32)  [unwired: 2 in, 2 out]
          n471 = Less?(x=w1170, y=227) -> (x < y?=w1167:bool)
          n472 = Or(x=w1167, y=w1166) -> (x .or. y?=w1165:bool)
        }
        n473 = local write "M11"(FALSE ("M11")) -> ()
        n474 = local write "M12"(TRUE ("M12")) -> ()
      }
    }
    n475 = case shown="True" w288 {
      frame False {
      }
      frame True {
        n476 = while {
          stop <- w1113 stop-if-true
          n477 = property on="vastago3 tapado" class="Bool (strict)"() -> ("Top"=w1124:i32)  [unwired: 2 in, 2 out]
          n478 = Subtract(x=w1124, y=1) -> (x-y=w1122:i32)
          n479 = property on="vastago3 tapado" class="Bool (strict)"("Top"=w1122) -> ()  [unwired: 2 in, 2 out]
          n480 = property on="vastago4 tapado" class="Bool (strict)"() -> ("Top"=w1121:i32)  [unwired: 2 in, 2 out]
          n481 = Subtract(x=w1121, y=2) -> (x-y=w1119:i32)
          n482 = property on="vastago4 tapado" class="Bool (strict)"("Top"=w1119) -> ()  [unwired: 2 in, 2 out]
          n483 = Wait (ms)(milliseconds to wait=u32 0) -> ()  [unwired: 1 out]
          n484 = local read "RESET"() -> (w1114:bool)
          n485 = property on="vastago3 tapado" class="Bool (strict)"() -> ("Top"=w1118:i32)  [unwired: 2 in, 2 out]
          n486 = Less?(x=w1118, y=207) -> (x < y?=w1115:bool)
          n487 = Or(x=w1115, y=w1114) -> (x .or. y?=w1113:bool)
        }
        n488 = local write "M14"(FALSE ("M14")) -> ()
        n489 = local write "M15"(TRUE ("M15")) -> ()
      }
    }
    n490 = case shown="True" w278 {
      frame False {
      }
      frame True {
        n491 = while {
          stop <- w1082 stop-if-true
          n492 = property on="BALANZA1" class="Bool (strict)"() -> ("Top"=w1090:i32)  [unwired: 2 in, 2 out]
          n493 = Subtract(x=w1090, y=2) -> (x-y=w1088:i32)
          n494 = property on="BALANZA1" class="Bool (strict)"("Top"=w1088) -> ()  [unwired: 2 in, 2 out]
          n495 = Wait (ms)(milliseconds to wait=u32 0) -> ()  [unwired: 1 out]
          n496 = local read "RESET"() -> (w1085:bool)
          n497 = property on="BALANZA1" class="Bool (strict)"() -> ("Top"=w1087:i32)  [unwired: 2 in, 2 out]
          n498 = Less?(x=w1087, y=109) -> (x < y?=w1084:bool)
          n499 = Or(x=w1084, y=w1085) -> (x .or. y?=w1082:bool)
        }
        n500 = local write "M16"(FALSE ("M16")) -> ()
        n501 = local write "M17"(TRUE ("M17")) -> ()
      }
    }
    n502 = case shown="True" w273 {
      frame False {
      }
      frame True {
        n503 = while {
          stop <- w1068 stop-if-true
          n504 = property on="BALANZA1" class="Bool (strict)"() -> ("Top"=w1079:i32)  [unwired: 2 in, 2 out]
          n505 = Subtract(x=w1079, y=2) -> (x-y=w1077:i32)
          n506 = property on="BALANZA1" class="Bool (strict)"("Top"=w1077) -> ()  [unwired: 2 in, 2 out]
          n507 = property on="TAPA NEUTRO" class="Bool (strict)"() -> ("Top"=w1073:i32)  [unwired: 2 in, 2 out]
          n508 = Subtract(x=w1073, y=2) -> (x-y=w1072:i32)
          n509 = property on="TAPA NEUTRO" class="Bool (strict)"("Top"=w1072) -> ()  [unwired: 2 in, 2 out]
          n510 = Wait (ms)(milliseconds to wait=u32 0) -> ()  [unwired: 1 out]
          n511 = local read "RESET"() -> (w1069:bool)
          n512 = property on="TAPA NEUTRO" class="Bool (strict)"() -> ("Top"=w1075:i32)  [unwired: 2 in, 2 out]
          n513 = Less?(x=w1075, y=16) -> (x < y?=w1071:bool)
          n514 = Or(x=w1071, y=w1069) -> (x .or. y?=w1068:bool)
        }
        n515 = local write "M17"(FALSE ("M17")) -> ()
        n516 = local write "M18"(TRUE ("M18")) -> ()
      }
    }
    n517 = case shown="True" w268 {
      frame False {
      }
      frame True {
        n518 = while {
          stop <- w1057 stop-if-true
          n519 = property on="BALANZA1" class="Bool (strict)"() -> ("Top"=w1065:i32)  [unwired: 2 in, 2 out]
          n520 = Add(x=w1065, y=2) -> (x+y=w1063:i32)
          n521 = property on="BALANZA1" class="Bool (strict)"("Top"=w1063) -> ()  [unwired: 2 in, 2 out]
          n522 = Wait (ms)(milliseconds to wait=u32 0) -> ()  [unwired: 1 out]
          n523 = local read "RESET"() -> (w1058:bool)
          n524 = property on="BALANZA1" class="Bool (strict)"() -> ("Top"=w1062:i32)  [unwired: 2 in, 2 out]
          n525 = Greater?(x=w1062, y=145) -> (0:w1059:bool)
          n526 = Or(x=w1059, y=w1058) -> (x .or. y?=w1057:bool)
        }
        n527 = local write "M18"(FALSE ("M18")) -> ()
        n528 = local write "M19"(TRUE ("M19")) -> ()
        n529 = local write "ANALIZANDO\nCC"(TRUE ("ANALIZANDO\nCC")) -> ()
      }
    }
    n530 = case shown="True" w260 {
      frame False {
      }
      frame True {
        n531 = while {
          stop <- w1020 stop-if-true
          n532 = property on="balanza2" class="Bool (strict)"() -> ("Left"=w1031:i32)  [unwired: 2 in, 2 out]
          n533 = Subtract(x=w1031, y=3) -> (x-y=w1029:i32)
          n534 = property on="balanza2" class="Bool (strict)"("Left"=w1029) -> ()  [unwired: 2 in, 2 out]
          n535 = property on="TAPA TARRO ROJO" class="Bool (strict)"() -> ("Left"=w1028:i32)  [unwired: 2 in, 2 out]
          n536 = Subtract(x=w1028, y=3) -> (x-y=w1026:i32)
          n537 = property on="TAPA TARRO ROJO" class="Bool (strict)"("Left"=w1026) -> ()  [unwired: 2 in, 2 out]
          n538 = Wait (ms)(milliseconds to wait=u32 0) -> ()  [unwired: 1 out]
          n539 = local read "RESET"() -> (w1021:bool)
          n540 = property on="balanza2" class="Bool (strict)"() -> ("Left"=w1024:i32)  [unwired: 2 in, 2 out]
          n541 = Less?(x=w1024, y=900) -> (x < y?=w1022:bool)
          n542 = Or(x=w1022, y=w1021) -> (x .or. y?=w1020:bool)
        }
        n543 = local write "M20"(FALSE ("M21")) -> ()
        n544 = local write "M21"(TRUE ("M22")) -> ()
      }
    }
    n545 = case shown="True" w255 {
      frame False {
      }
      frame True {
        n546 = while {
          stop <- w1006 stop-if-true
          n547 = property on="TAPA TARRO ROJO" class="Bool (strict)"() -> ("Left"=w1017:i32)  [unwired: 2 in, 2 out]
          n548 = Subtract(x=w1017, y=3) -> (x-y=w1015:i32)
          n549 = property on="TAPA TARRO ROJO" class="Bool (strict)"("Left"=w1015) -> ()  [unwired: 2 in, 2 out]
          n550 = property on="balanza2" class="Bool (strict)"() -> ("Left"=w1014:i32)  [unwired: 2 in, 2 out]
          n551 = Add(x=w1014, y=3) -> (x+y=w1012:i32)
          n552 = property on="balanza2" class="Bool (strict)"("Left"=w1012) -> ()  [unwired: 2 in, 2 out]
          n553 = Wait (ms)(milliseconds to wait=u32 0) -> ()  [unwired: 1 out]
          n554 = local read "RESET"() -> (w1007:bool)
          n555 = property on="balanza2" class="Bool (strict)"() -> ("Left"=w1010:i32)  [unwired: 2 in, 2 out]
          n556 = Greater?(x=w1010, y=977) -> (0:w1008:bool)
          n557 = Or(x=w1008, y=w1007) -> (x .or. y?=w1006:bool)
        }
        n558 = local write "M22"(TRUE ("M23")) -> ()
        n559 = local write "M21"(FALSE ("M22")) -> ()
      }
    }
    n560 = case shown="True" w250 {
      frame False {
      }
      frame True {
        n561 = while {
          stop <- w995 stop-if-true
          n562 = property on="TAPA TARRO ROJO" class="Bool (strict)"() -> ("Left"=w1003:i32)  [unwired: 2 in, 2 out]
          n563 = Subtract(x=w1003, y=3) -> (x-y=w1001:i32)
          n564 = property on="TAPA TARRO ROJO" class="Bool (strict)"("Left"=w1001) -> ()  [unwired: 2 in, 2 out]
          n565 = Wait (ms)(milliseconds to wait=u32 0) -> ()  [unwired: 1 out]
          n566 = local read "RESET"() -> (w996:bool)
          n567 = property on="TAPA TARRO ROJO" class="Bool (strict)"() -> ("Left"=w999:i32)  [unwired: 2 in, 2 out]
          n568 = Less?(x=w999, y=426) -> (x < y?=w998:bool)
          n569 = Or(x=w998, y=w996) -> (x .or. y?=w995:bool)
        }
        n570 = local write "M23"(TRUE ("M24")) -> ()
        n571 = local write "M22"(FALSE ("M23")) -> ()
      }
    }
    n572 = case shown="True" w245 {
      frame False {
      }
      frame True {
        n573 = while {
          stop <- w981 stop-if-true
          n574 = property on="VASTAGO MODULO6" class="Bool (strict)"() -> ("Top"=w991:i32)  [unwired: 2 in, 2 out]
          n575 = Add(x=w991, y=2) -> (x+y=w989:i32)
          n576 = property on="VASTAGO MODULO6" class="Bool (strict)"("Top"=w989) -> ()  [unwired: 2 in, 2 out]
          n577 = property on="TAPA TARRO ROJO" class="Bool (strict)"() -> ("Top"=w988:i32)  [unwired: 2 in, 2 out]
          n578 = Add(x=w988, y=2) -> (x+y=w986:i32)
          n579 = property on="TAPA TARRO ROJO" class="Bool (strict)"("Top"=w986) -> ()  [unwired: 2 in, 2 out]
          n580 = Wait (ms)(milliseconds to wait=u32 0) -> ()  [unwired: 1 out]
          n581 = local read "RESET"() -> (w982:bool)
          n582 = property on="VASTAGO MODULO6" class="Bool (strict)"() -> ("Top"=w985:i32)  [unwired: 2 in, 2 out]
          n583 = Greater?(x=w985, y=55) -> (0:w984:bool)
          n584 = Or(x=w984, y=w982) -> (x .or. y?=w981:bool)
        }
        n585 = local write "M23"(FALSE ("M24")) -> ()
        n586 = local write "M24"(TRUE ("M25")) -> ()
        n587 = Wait (ms)(milliseconds to wait=u32 1000) -> ()  [unwired: 1 out]
      }
    }
    n588 = case shown="True" w240 {
      frame False {
      }
      frame True {
        n589 = local read "FINALIZADOS\nROJOS"() -> (w968:dbl)
        n590 = Increment(x=w968) -> (x+1=w967:dbl)
        n591 = local write "FINALIZADOS\nROJOS"(w967) -> ()
        n592 = while {
          stop <- w969 stop-if-true
          n593 = property on="VASTAGO MODULO6" class="Bool (strict)"() -> ("Top"=w977:i32)  [unwired: 2 in, 2 out]
          n594 = Subtract(x=w977, y=1) -> (x-y=w975:i32)
          n595 = property on="VASTAGO MODULO6" class="Bool (strict)"("Top"=w975) -> ()  [unwired: 2 in, 2 out]
          n596 = Wait (ms)(milliseconds to wait=u32 0) -> ()  [unwired: 1 out]
          n597 = local read "RESET"() -> (w970:bool)
          n598 = property on="VASTAGO MODULO6" class="Bool (strict)"() -> ("Top"=w973:i32)  [unwired: 2 in, 2 out]
          n599 = Less?(x=w973, y=-10) -> (x < y?=w971:bool)
          n600 = Or(x=w971, y=w970) -> (x .or. y?=w969:bool)
        }
        n601 = local write "M25"(TRUE ("M30")) -> ()
        n602 = local write "M24"(FALSE ("M25")) -> ()
        n603 = local write "PESO\nSI"(FALSE ("PESO\nSI")) -> ()
        n604 = local write "ROJO"(FALSE ("ROJO")) -> ()
      }
    }
    n605 = case shown="True" w235 {
      frame False {
      }
      frame True {
        n606 = property on="TAPA TARRO ROJO" class="Bool (strict)"("Visible"=FALSE) -> ()  [unwired: 2 in, 2 out]
        n607 = local write "M25"(FALSE ("M30")) -> ()
        n608 = local write "reinicio"(TRUE ("reinicio")) -> ()
      }
    }
    n609 = case shown="True" w223 {
      frame False {
      }
      frame True {
        n610 = while {
          stop <- w926 stop-if-true
          n611 = property on="TAPA AZUL" class="Bool (strict)"() -> ("Left"=w937:i32)  [unwired: 2 in, 2 out]
          n612 = Subtract(x=w937, y=3) -> (x-y=w935:i32)
          n613 = property on="TAPA AZUL" class="Bool (strict)"("Left"=w935) -> ()  [unwired: 2 in, 2 out]
          n614 = property on="balanza2" class="Bool (strict)"() -> ("Left"=w934:i32)  [unwired: 2 in, 2 out]
          n615 = Subtract(x=w934, y=3) -> (x-y=w932:i32)
          n616 = property on="balanza2" class="Bool (strict)"("Left"=w932) -> ()  [unwired: 2 in, 2 out]
          n617 = Wait (ms)(milliseconds to wait=u32 0) -> ()  [unwired: 1 out]
          n618 = property on="balanza2" class="Bool (strict)"() -> ("Left"=w930:i32)  [unwired: 2 in, 2 out]
          n619 = local read "RESET"() -> (w927:bool)
          n620 = Less?(x=w930, y=900) -> (x < y?=w928:bool)
          n621 = Or(x=w928, y=w927) -> (x .or. y?=w926:bool)
        }
        n622 = local write "M26"(FALSE ("M26")) -> ()
        n623 = local write "M27"(TRUE ("M27")) -> ()
      }
    }
    n624 = case shown="True" w218 {
      frame False {
      }
      frame True {
        n625 = while {
          stop <- w912 stop-if-true
          n626 = property on="balanza2" class="Bool (strict)"() -> ("Left"=w922:i32)  [unwired: 2 in, 2 out]
          n627 = Add(x=w922, y=3) -> (x+y=w923:i32)
          n628 = property on="balanza2" class="Bool (strict)"("Left"=w923) -> ()  [unwired: 2 in, 2 out]
          n629 = property on="TAPA AZUL" class="Bool (strict)"() -> ("Left"=w919:i32)  [unwired: 2 in, 2 out]
          n630 = Subtract(x=w919, y=3) -> (x-y=w920:i32)
          n631 = property on="TAPA AZUL" class="Bool (strict)"("Left"=w920) -> ()  [unwired: 2 in, 2 out]
          n632 = Wait (ms)(milliseconds to wait=u32 0) -> ()  [unwired: 1 out]
          n633 = local read "RESET"() -> (w913:bool)
          n634 = property on="balanza2" class="Bool (strict)"() -> ("Left"=w916:i32)  [unwired: 2 in, 2 out]
          n635 = Greater?(x=w916, y=977) -> (0:w914:bool)
          n636 = Or(x=w914, y=w913) -> (x .or. y?=w912:bool)
        }
        n637 = local write "M28"(TRUE ("M28")) -> ()
        n638 = local write "M27"(FALSE ("M27")) -> ()
      }
    }
    n639 = case shown="True" w213 {
      frame False {
      }
      frame True {
        n640 = while {
          stop <- w901 stop-if-true
          n641 = property on="TAPA AZUL" class="Bool (strict)"() -> ("Left"=w909:i32)  [unwired: 2 in, 2 out]
          n642 = Subtract(x=w909, y=3) -> (x-y=w907:i32)
          n643 = property on="TAPA AZUL" class="Bool (strict)"("Left"=w907) -> ()  [unwired: 2 in, 2 out]
          n644 = Wait (ms)(milliseconds to wait=u32 0) -> ()  [unwired: 1 out]
          n645 = local read "RESET"() -> (w902:bool)
          n646 = property on="TAPA AZUL" class="Bool (strict)"() -> ("Left"=w905:i32)  [unwired: 2 in, 2 out]
          n647 = Less?(x=w905, y=426) -> (x < y?=w903:bool)
          n648 = Or(x=w903, y=w902) -> (x .or. y?=w901:bool)
        }
        n649 = local write "M28"(FALSE ("M28")) -> ()
        n650 = local write "M29"(TRUE ("M29")) -> ()
      }
    }
    n651 = case shown="True" w203 {
      frame False {
      }
      frame True {
        n652 = while {
          stop <- w867 stop-if-true
          n653 = property on="TAPA AZUL" class="Bool (strict)"() -> ("Top"=w878:i32)  [unwired: 2 in, 2 out]
          n654 = Add(x=w878, y=2) -> (x+y=w876:i32)
          n655 = property on="TAPA AZUL" class="Bool (strict)"("Top"=w876) -> ()  [unwired: 2 in, 2 out]
          n656 = property on="VASTAGO MODULO6" class="Bool (strict)"() -> ("Top"=w875:i32)  [unwired: 2 in, 2 out]
          n657 = Add(x=w875, y=2) -> (x+y=w873:i32)
          n658 = property on="VASTAGO MODULO6" class="Bool (strict)"("Top"=w873) -> ()  [unwired: 2 in, 2 out]
          n659 = Wait (ms)(milliseconds to wait=u32 0) -> ()  [unwired: 1 out]
          n660 = local read "RESET"() -> (w868:bool)
          n661 = property on="VASTAGO MODULO6" class="Bool (strict)"() -> ("Top"=w871:i32)  [unwired: 2 in, 2 out]
          n662 = Greater?(x=w871, y=55) -> (0:w869:bool)
          n663 = Or(x=w869, y=w868) -> (x .or. y?=w867:bool)
        }
        n664 = local write "M30"(FALSE ("M30")) -> ()
        n665 = local write "M31"(TRUE ("M31")) -> ()
      }
    }
    n666 = case shown="True" w188 {
      frame False {
      }
      frame True {
        n667 = local write "M33"(FALSE ("M33")) -> ()
        n668 = property on="TAPA AZUL" class="Bool (strict)"("Visible"=FALSE) -> ()  [unwired: 2 in, 2 out]
        n669 = local write "reinicio"(TRUE ("reinicio")) -> ()
      }
    }
    n670 = case shown="True" w179 {
      frame False {
      }
      frame True {
        n671 = while {
          stop <- w790 stop-if-true
          n672 = property on="TAPA NOCOLOR" class="Bool (strict)"() -> ("Left"=w801:i32)  [unwired: 2 in, 2 out]
          n673 = Subtract(x=w801, y=6) -> (x-y=w799:i32)
          n674 = property on="TAPA NOCOLOR" class="Bool (strict)"("Left"=w799) -> ()  [unwired: 2 in, 2 out]
          n675 = property on="balanza2" class="Bool (strict)"() -> ("Left"=w798:i32)  [unwired: 2 in, 2 out]
          n676 = Subtract(x=w798, y=6) -> (x-y=w796:i32)
          n677 = property on="balanza2" class="Bool (strict)"("Left"=w796) -> ()  [unwired: 2 in, 2 out]
          n678 = Wait (ms)(milliseconds to wait=u32 0) -> ()  [unwired: 1 out]
          n679 = local read "RESET"() -> (w791:bool)
          n680 = property on="balanza2" class="Bool (strict)"() -> ("Left"=w794:i32)  [unwired: 2 in, 2 out]
          n681 = Less?(x=w794, y=900) -> (x < y?=w792:bool)
          n682 = Or(x=w792, y=w791) -> (x .or. y?=w790:bool)
        }
        n683 = local write "M34"(FALSE ("M34")) -> ()
        n684 = local write "M35"(TRUE ("M35")) -> ()
      }
    }
    n685 = case shown="True" w174 {
      frame False {
      }
      frame True {
        n686 = while {
          stop <- w776 stop-if-true
          n687 = property on="balanza2" class="Bool (strict)"() -> ("Left"=w786:i32)  [unwired: 2 in, 2 out]
          n688 = Add(x=w786, y=6) -> (x+y=w787:i32)
          n689 = property on="balanza2" class="Bool (strict)"("Left"=w787) -> ()  [unwired: 2 in, 2 out]
          n690 = property on="TAPA NOCOLOR" class="Bool (strict)"() -> ("Left"=w784:i32)  [unwired: 2 in, 2 out]
          n691 = Subtract(x=w784, y=6) -> (x-y=w782:i32)
          n692 = property on="TAPA NOCOLOR" class="Bool (strict)"("Left"=w782) -> ()  [unwired: 2 in, 2 out]
          n693 = Wait (ms)(milliseconds to wait=u32 0) -> ()  [unwired: 1 out]
          n694 = local read "RESET"() -> (w777:bool)
          n695 = property on="balanza2" class="Bool (strict)"() -> ("Left"=w780:i32)  [unwired: 2 in, 2 out]
          n696 = Greater?(x=w780, y=977) -> (0:w778:bool)
          n697 = Or(x=w778, y=w777) -> (x .or. y?=w776:bool)
        }
        n698 = local write "M35"(FALSE ("M35")) -> ()
        n699 = local write "M36"(TRUE ("M36")) -> ()
      }
    }
    n700 = case shown="True" w167 {
      frame False {
      }
      frame True {
        n701 = while {
          stop <- w765 stop-if-true
          n702 = property on="TAPA NOCOLOR" class="Bool (strict)"() -> ("Left"=w773:i32)  [unwired: 2 in, 2 out]
          n703 = Subtract(x=w773, y=6) -> (x-y=w771:i32)
          n704 = property on="TAPA NOCOLOR" class="Bool (strict)"("Left"=w771) -> ()  [unwired: 2 in, 2 out]
          n705 = Wait (ms)(milliseconds to wait=u32 0) -> ()  [unwired: 1 out]
          n706 = local read "RESET"() -> (w766:bool)
          n707 = property on="TAPA NOCOLOR" class="Bool (strict)"() -> ("Left"=w769:i32)  [unwired: 2 in, 2 out]
          n708 = Less?(x=w769, y=737) -> (x < y?=w767:bool)
          n709 = Or(x=w767, y=w766) -> (x .or. y?=w765:bool)
        }
        n710 = local write "M37"(TRUE ("M37")) -> ()
        n711 = local write "M36"(FALSE ("M36")) -> ()
      }
    }
    n712 = case shown="True" w132 {
      frame False {
      }
      frame True {
        n713 = property on="PINZA ABIERTA" class="Bool (strict)"("Visible"=FALSE) -> ()  [unwired: 2 in, 2 out]
        n714 = property on="VASTAGO RECHAZO" class="Bool (strict)"("Visible"=FALSE) -> ()  [unwired: 2 in, 2 out]
        n715 = local write "M43"(FALSE ("M43")) -> ()
        n716 = property on="TARRO NOCOLOR" class="Bool (strict)"("Visible"=FALSE) -> ()  [unwired: 2 in, 2 out]
        n717 = property on="CILINDRO RECHAZO" class="Bool (strict)"("Visible"=FALSE) -> ()  [unwired: 2 in, 2 out]
        n718 = property on="CILINDRO RECHAZO1" class="Bool (strict)"("Visible"=FALSE) -> ()  [unwired: 2 in, 2 out]
        n719 = property on="TAPA NOCOLOR" class="Bool (strict)"("Visible"=FALSE) -> ()  [unwired: 2 in, 2 out]
        n720 = property on="ESTRUCTURA RECHAZO" class="Bool (strict)"("Visible"=FALSE) -> ()  [unwired: 2 in, 2 out]
        n721 = property on="DEPOSITO NOCOLOR" class="Bool (strict)"("Visible"=FALSE) -> ()  [unwired: 2 in, 2 out]
        n722 = property on="DEPOSITO NOPESO" class="Bool (strict)"("Visible"=FALSE) -> ()  [unwired: 2 in, 2 out]
        n723 = local write "reinicio"(TRUE ("reinicio")) -> ()
      }
    }
    n724 = case shown="True" w117 {
      frame False {
      }
      frame True {
        n725 = while {
          stop <- w566 stop-if-true
          n726 = property on="TAPA NOPESO" class="Bool (strict)"() -> ("Left"=w577:i32)  [unwired: 2 in, 2 out]
          n727 = Subtract(x=w577, y=6) -> (x-y=w575:i32)
          n728 = property on="TAPA NOPESO" class="Bool (strict)"("Left"=w575) -> ()  [unwired: 2 in, 2 out]
          n729 = property on="balanza2" class="Bool (strict)"() -> ("Left"=w574:i32)  [unwired: 2 in, 2 out]
          n730 = Subtract(x=w574, y=6) -> (x-y=w572:i32)
          n731 = property on="balanza2" class="Bool (strict)"("Left"=w572) -> ()  [unwired: 2 in, 2 out]
          n732 = Wait (ms)(milliseconds to wait=u32 0) -> ()  [unwired: 1 out]
          n733 = local read "RESET"() -> (w567:bool)
          n734 = property on="balanza2" class="Bool (strict)"() -> ("Left"=w570:i32)  [unwired: 2 in, 2 out]
          n735 = Less?(x=w570, y=900) -> (x < y?=w568:bool)
          n736 = Or(x=w568, y=w567) -> (x .or. y?=w566:bool)
        }
        n737 = local write "M44"(FALSE ("M44")) -> ()
        n738 = local write "M45"(TRUE ("M45")) -> ()
      }
    }
    n739 = case shown="True" w112 {
      frame False {
      }
      frame True {
        n740 = while {
          stop <- w552 stop-if-true
          n741 = property on="TAPA NOPESO" class="Bool (strict)"() -> ("Left"=w563:i32)  [unwired: 2 in, 2 out]
          n742 = Subtract(x=w563, y=6) -> (x-y=w561:i32)
          n743 = property on="TAPA NOPESO" class="Bool (strict)"("Left"=w561) -> ()  [unwired: 2 in, 2 out]
          n744 = property on="balanza2" class="Bool (strict)"() -> ("Left"=w560:i32)  [unwired: 2 in, 2 out]
          n745 = Add(x=w560, y=6) -> (x+y=w558:i32)
          n746 = property on="balanza2" class="Bool (strict)"("Left"=w558) -> ()  [unwired: 2 in, 2 out]
          n747 = Wait (ms)(milliseconds to wait=u32 0) -> ()  [unwired: 1 out]
          n748 = local read "RESET"() -> (w553:bool)
          n749 = property on="balanza2" class="Bool (strict)"() -> ("Left"=w556:i32)  [unwired: 2 in, 2 out]
          n750 = Greater?(x=w556, y=977) -> (0:w554:bool)
          n751 = Or(x=w554, y=w553) -> (x .or. y?=w552:bool)
        }
        n752 = local write "M45"(FALSE ("M45")) -> ()
        n753 = local write "M46"(TRUE ("M46")) -> ()
      }
    }
    n754 = case shown="True" w107 {
      frame False {
      }
      frame True {
        n755 = while {
          stop <- w541 stop-if-true
          n756 = property on="TAPA NOPESO" class="Bool (strict)"() -> ("Left"=w549:i32)  [unwired: 2 in, 2 out]
          n757 = Subtract(x=w549, y=6) -> (x-y=w547:i32)
          n758 = property on="TAPA NOPESO" class="Bool (strict)"("Left"=w547) -> ()  [unwired: 2 in, 2 out]
          n759 = Wait (ms)(milliseconds to wait=u32 0) -> ()  [unwired: 1 out]
          n760 = local read "RESET"() -> (w542:bool)
          n761 = property on="TAPA NOPESO" class="Bool (strict)"() -> ("Left"=w545:i32)  [unwired: 2 in, 2 out]
          n762 = Less?(x=w545, y=737) -> (x < y?=w543:bool)
          n763 = Or(x=w543, y=w542) -> (x .or. y?=w541:bool)
        }
        n764 = local write "M46"(FALSE ("M46")) -> ()
        n765 = local write "M47"(TRUE ("M47")) -> ()
      }
    }
    n766 = case shown="True" w70 {
      frame False {
      }
      frame True {
        n767 = property on="PINZA ABIERTA" class="Bool (strict)"("Visible"=FALSE) -> ()  [unwired: 2 in, 2 out]
        n768 = property on="VASTAGO RECHAZO" class="Bool (strict)"("Visible"=FALSE) -> ()  [unwired: 2 in, 2 out]
        n769 = property on="TAPA NOPESO" class="Bool (strict)"("Visible"=FALSE) -> ()  [unwired: 2 in, 2 out]
        n770 = property on="CILINDRO RECHAZO" class="Bool (strict)"("Visible"=FALSE) -> ()  [unwired: 2 in, 2 out]
        n771 = property on="CILINDRO RECHAZO1" class="Bool (strict)"("Visible"=FALSE) -> ()  [unwired: 2 in, 2 out]
        n772 = property on="TARRO NOPESO" class="Bool (strict)"("Visible"=FALSE) -> ()  [unwired: 2 in, 2 out]
        n773 = property on="ESTRUCTURA RECHAZO" class="Bool (strict)"("Visible"=FALSE) -> ()  [unwired: 2 in, 2 out]
        n774 = property on="DEPOSITO NOPESO" class="Bool (strict)"("Visible"=FALSE) -> ()  [unwired: 2 in, 2 out]
        n775 = property on="DEPOSITO NOCOLOR" class="Bool (strict)"("Visible"=FALSE) -> ()  [unwired: 2 in, 2 out]
        n776 = local write "reinicio"(TRUE ("reinicio")) -> ()
        n777 = local write "M54"(FALSE ("M54")) -> ()
      }
    }
    n778 = case shown="True" w183 {
      frame False {
      }
      frame True {
        n779 = property on="TAPA NEUTRO" class="Bool (strict)"("Visible"=FALSE) -> ()  [unwired: 2 in, 2 out]
        n780 = property on="TAPA NOCOLOR" class="Bool (strict)"("Visible"=TRUE) -> ()  [unwired: 2 in, 2 out]
        n781 = property on="ACTUADOR RECHAZO" class="Bool (strict)"("Top"=220 ("Position:Top")) -> ()  [unwired: 2 in, 2 out]
        n782 = property on="CILINDRO RECHAZO" class="Bool (strict)"("Left"=592 ("Position:Left")) -> ()  [unwired: 2 in, 2 out]
        n783 = property on="VASTAGO RECHAZO" class="Bool (strict)"("Top"=180 ("Position:Top")) -> ()  [unwired: 2 in, 2 out]
        n784 = property on="CILINDRO RECHAZO1" class="Bool (strict)"("Left"=620 ("Position:Left")) -> ()  [unwired: 2 in, 2 out]
        n785 = property on="VASTAGO RECHAZO" class="Bool (strict)"("Left"=614 ("Position:Left")) -> ()  [unwired: 2 in, 2 out]
        n786 = property on="TAPA NOCOLOR" class="Bool (strict)"("Left"=917 ("Position:Left")) -> ()  [unwired: 2 in, 2 out]
        n787 = property on="TAPA NOCOLOR" class="Bool (strict)"("Top"=14 ("Position:Top")) -> ()  [unwired: 2 in, 2 out]
        n788 = property on="PINZA CERRADA" class="Bool (strict)"("Left"=596 ("Position:Left")) -> ()  [unwired: 2 in, 2 out]
        n789 = property on="PINZA CERRADA" class="Bool (strict)"("Top"=316 ("Position:Top")) -> ()  [unwired: 2 in, 2 out]
        n790 = property on="PINZA ABIERTA" class="Bool (strict)"("Left"=587 ("Position:Left")) -> ()  [unwired: 2 in, 2 out]
        n791 = property on="PINZA ABIERTA" class="Bool (strict)"("Top"=313 ("Position:Top")) -> ()  [unwired: 2 in, 2 out]
        n792 = property on="TARRO NOCOLOR" class="Bool (strict)"("Left"=386 ("Position:Left")) -> ()  [unwired: 2 in, 2 out]
        n793 = property on="TARRO NOCOLOR" class="Bool (strict)"("Top"=409 ("Position:Top")) -> ()  [unwired: 2 in, 2 out]
        n794 = while {
          stop <- w821 stop-if-true
          n795 = property on="balanza2" class="Bool (strict)"() -> ("Left"=w829:i32)  [unwired: 2 in, 2 out]
          n796 = Subtract(x=w829, y=6) -> (x-y=w827:i32)
          n797 = property on="balanza2" class="Bool (strict)"("Left"=w827) -> ()  [unwired: 2 in, 2 out]
          n798 = Wait (ms)(milliseconds to wait=u32 0) -> ()  [unwired: 1 out]
          n799 = local read "RESET"() -> (w822:bool)
          n800 = property on="balanza2" class="Bool (strict)"() -> ("Left"=w825:i32)  [unwired: 2 in, 2 out]
          n801 = Less?(x=w825, y=965) -> (x < y?=w823:bool)
          n802 = Or(x=w823, y=w822) -> (x .or. y?=w821:bool)
        }
        n803 = local write "ANALIZANDO\nCC"(FALSE ("ANALIZANDO\nCC")) -> ()
        n804 = local write "NO \nCOLOR"(TRUE ("NO \nCOLOR")) -> ()
        n805 = local write "M19"(FALSE ("M19")) -> ()
        n806 = local write "M34"(TRUE ("M34")) -> ()
      }
    }
    n807 = case shown="True" w338 {
      frame False {
      }
      frame True {
        n808 = property on="cilindros tolva" class="Bool (strict)"("Visible"=TRUE) -> ()  [unwired: 2 in, 2 out]
        n809 = property on="perta tolva1" class="Bool (strict)"("Visible"=TRUE) -> ()  [unwired: 2 in, 2 out]
        n810 = property on="tarro vaciop1" class="Bool (strict)"("Visible"=TRUE) -> ()  [unwired: 2 in, 2 out]
        n811 = property on="dep superior" class="Bool (strict)"("Visible"=TRUE) -> ()  [unwired: 2 in, 2 out]
        n812 = property on="puerta tolva2" class="Bool (strict)"("Visible"=TRUE) -> ()  [unwired: 2 in, 2 out]
        n813 = property on="tolva vacia" class="Bool (strict)"("Visible"=TRUE) -> ()  [unwired: 2 in, 2 out]
        n814 = while {
          stop <- w1293 stop-if-true
          n815 = property on="PUERTA TOLVA" class="Bool (strict)"() -> ("Left"=w1304:i32)  [unwired: 2 in, 2 out]
          n816 = Add(x=w1304, y=1) -> (x+y=w1302:i32)
          n817 = property on="PUERTA TOLVA" class="Bool (strict)"("Left"=w1302) -> ()  [unwired: 2 in, 2 out]
          n818 = property on="perta tolva1" class="Bool (strict)"() -> ("Left"=w1298:i32)  [unwired: 2 in, 2 out]
          n819 = Subtract(x=w1298, y=1) -> (x-y=w1296:i32)
          n820 = property on="perta tolva1" class="Bool (strict)"("Left"=w1296) -> ()  [unwired: 2 in, 2 out]
          n821 = Wait (ms)(milliseconds to wait=u32 0) -> ()  [unwired: 1 out]
          n822 = property on="PUERTA TOLVA" class="Bool (strict)"() -> ("Left"=w1301:i32)  [unwired: 2 in, 2 out]
          n823 = local read "RESET"() -> (w1294:bool)
          n824 = Greater?(x=w1301, y=950) -> (0:w1299:bool)
          n825 = Or(x=w1299, y=w1294) -> (x .or. y?=w1293:bool)
        }
        n826 = local write "M4"(FALSE ("M4")) -> ()
        n827 = local write "M5"(TRUE ("M5")) -> ()
      }
    }
    n828 = case shown="True" w318 {
      frame False {
      }
      frame True {
        n829 = property on="TARRO VACIO" class="Bool (strict)"("Visible"=FALSE) -> ()  [unwired: 2 in, 2 out]
        n830 = property on="CAJA LLENA" class="Bool (strict)"("Visible"=TRUE) -> ()  [unwired: 2 in, 2 out]
        n831 = property on="tarro vaciop1" class="Bool (strict)"("Visible"=FALSE) -> ()  [unwired: 2 in, 2 out]
        n832 = property on="tolva vacia" class="Bool (strict)"("Visible"=FALSE) -> ()  [unwired: 2 in, 2 out]
        n833 = property on="dep inferior" class="Bool (strict)"("Visible"=FALSE) -> ()  [unwired: 2 in, 2 out]
        n834 = property on="dep superior" class="Bool (strict)"("Visible"=FALSE) -> ()  [unwired: 2 in, 2 out]
        n835 = property on="cilindros tolva" class="Bool (strict)"("Visible"=FALSE) -> ()  [unwired: 2 in, 2 out]
        n836 = property on="puerta tolva2" class="Bool (strict)"("Visible"=FALSE) -> ()  [unwired: 2 in, 2 out]
        n837 = property on="perta tolva1" class="Bool (strict)"("Visible"=FALSE) -> ()  [unwired: 2 in, 2 out]
        n838 = property on="tarro llenop" class="Bool (strict)"("Visible"=FALSE) -> ()  [unwired: 2 in, 2 out]
        n839 = while {
          stop <- w1236 stop-if-true
          n840 = property on="CAJA LLENA" class="Bool (strict)"() -> ("Top"=w1243:i32)  [unwired: 2 in, 2 out]
          n841 = Subtract(x=w1243, y=2) -> (x-y=w1241:i32)
          n842 = property on="CAJA LLENA" class="Bool (strict)"("Top"=w1241) -> ()  [unwired: 2 in, 2 out]
          n843 = Wait (ms)(milliseconds to wait=u32 0) -> ()  [unwired: 1 out]
          n844 = local read "RESET"() -> (w1237:bool)
          n845 = property on="CAJA LLENA" class="Bool (strict)"() -> ("Top"=w1240:i32)  [unwired: 2 in, 2 out]
          n846 = Less?(x=w1240, y=97) -> (x < y?=w1238:bool)
          n847 = Or(x=w1238, y=w1237) -> (x .or. y?=w1236:bool)
        }
        n848 = local write "M8"(FALSE ("M8")) -> ()
        n849 = local write "M9"(TRUE ("M9")) -> ()
      }
    }
    n850 = case shown="True" w293 {
      frame False {
      }
      frame True {
        n851 = while {
          stop <- w1127 stop-if-true
          n852 = property on="tapa neutrop" class="Bool (strict)"() -> ("Top"=w1141:i32)  [unwired: 2 in, 2 out]
          n853 = Add(x=w1141, y=2) -> (x+y=w1139:i32)
          n854 = property on="tapa neutrop" class="Bool (strict)"("Top"=w1139) -> ()  [unwired: 2 in, 2 out]
          n855 = property on="vastago3 tapado" class="Bool (strict)"() -> ("Top"=w1138:i32)  [unwired: 2 in, 2 out]
          n856 = Add(x=w1138, y=1) -> (x+y=w1136:i32)
          n857 = property on="vastago3 tapado" class="Bool (strict)"("Top"=w1136) -> ()  [unwired: 2 in, 2 out]
          n858 = property on="vastago4 tapado" class="Bool (strict)"() -> ("Top"=w1135:i32)  [unwired: 2 in, 2 out]
          n859 = Add(x=w1135, y=2) -> (x+y=w1133:i32)
          n860 = property on="vastago4 tapado" class="Bool (strict)"("Top"=w1133) -> ()  [unwired: 2 in, 2 out]
          n861 = Wait (ms)(milliseconds to wait=u32 0) -> ()  [unwired: 1 out]
          n862 = local read "RESET"() -> (w1128:bool)
          n863 = property on="tapa neutrop" class="Bool (strict)"() -> ("Top"=w1132:i32)  [unwired: 2 in, 2 out]
          n864 = Greater?(x=w1132, y=367) -> (0:w1129:bool)
          n865 = Or(x=w1129, y=w1128) -> (x .or. y?=w1127:bool)
        }
        n866 = local write "M13"(FALSE ("M13")) -> ()
        n867 = local write "M14"(TRUE ("M14")) -> ()
      }
    }
    n868 = case shown="True" w283 {
      frame False {
      }
      frame True {
        n869 = property on="estructura tapado" class="Bool (strict)"("Visible"=FALSE) -> ()  [unwired: 2 in, 2 out]
        n870 = property on="tapa neutrop" class="Bool (strict)"("Visible"=FALSE) -> ()  [unwired: 2 in, 2 out]
        n871 = property on="vastago1 tapado" class="Bool (strict)"("Visible"=FALSE) -> ()  [unwired: 2 in, 2 out]
        n872 = property on="cilindro1 tapado" class="Bool (strict)"("Visible"=FALSE) -> ()  [unwired: 2 in, 2 out]
        n873 = property on="vastago2 tapado" class="Bool (strict)"("Visible"=FALSE) -> ()  [unwired: 2 in, 2 out]
        n874 = property on="cilindro2 tapado" class="Bool (strict)"("Visible"=FALSE) -> ()  [unwired: 2 in, 2 out]
        n875 = property on="vastago3 tapado" class="Bool (strict)"("Visible"=FALSE) -> ()  [unwired: 2 in, 2 out]
        n876 = property on="cilindro3 tapado" class="Bool (strict)"("Visible"=FALSE) -> ()  [unwired: 2 in, 2 out]
        n877 = property on="vastago4 tapado" class="Bool (strict)"("Visible"=FALSE) -> ()  [unwired: 2 in, 2 out]
        n878 = while {
          stop <- w1102 stop-if-true
          n879 = property on="TAPA NEUTRO" class="Bool (strict)"() -> ("Top"=w1110:i32)  [unwired: 2 in, 2 out]
          n880 = Subtract(x=w1110, y=1) -> (x-y=w1108:i32)
          n881 = property on="TAPA NEUTRO" class="Bool (strict)"("Top"=w1108) -> ()  [unwired: 2 in, 2 out]
          n882 = Wait (ms)(milliseconds to wait=u32 0) -> ()  [unwired: 1 out]
          n883 = local read "RESET"() -> (w1104:bool)
          n884 = property on="TAPA NEUTRO" class="Bool (strict)"() -> ("Top"=w1107:i32)  [unwired: 2 in, 2 out]
          n885 = Less?(x=w1107, y=67) -> (x < y?=w1105:bool)
          n886 = Or(x=w1105, y=w1104) -> (x .or. y?=w1102:bool)
        }
        n887 = local write "M15"(FALSE ("M15")) -> ()
        n888 = local write "M16"(TRUE ("M16")) -> ()
      }
    }
    n889 = case shown="True" w263 {
      frame False {
      }
      frame True {
        n890 = property on="TAPA NEUTRO" class="Bool (strict)"("Visible"=FALSE) -> ()  [unwired: 2 in, 2 out]
        n891 = property on="TAPA TARRO ROJO" class="Bool (strict)"("Visible"=TRUE) -> ()  [unwired: 2 in, 2 out]
        n892 = property on="TAPA TARRO ROJO" class="Bool (strict)"("Left"=916 ("Position:Left")) -> ()  [unwired: 2 in, 2 out]
        n893 = property on="TAPA TARRO ROJO" class="Bool (strict)"("Top"=14 ("Position:Top")) -> ()  [unwired: 2 in, 2 out]
        n894 = property on="CILINDRO MODULO6" class="Bool (strict)"("Left"=376 ("Position:Left")) -> ()  [unwired: 2 in, 2 out]
        n895 = property on="VASTAGO MODULO6" class="Bool (strict)"("Left"=385 ("Position:Left")) -> ()  [unwired: 2 in, 2 out]
        n896 = property on="VASTAGO MODULO6" class="Bool (strict)"("Top"=-11 ("Position:Top")) -> ()  [unwired: 2 in, 2 out]
        n897 = property on="MODULO6" class="Bool (strict)"("Left"=378 ("Position:Left")) -> ()  [unwired: 2 in, 2 out]
        n898 = while {
          stop <- w1048 stop-if-true
          n899 = property on="balanza2" class="Bool (strict)"() -> ("Left"=w1053:i32)  [unwired: 2 in, 2 out]
          n900 = Subtract(x=w1053, y=3) -> (x-y=w1051:i32)
          n901 = property on="balanza2" class="Bool (strict)"("Left"=w1051) -> ()  [unwired: 2 in, 2 out]
          n902 = Wait (ms)(milliseconds to wait=u32 0) -> ()  [unwired: 1 out]
          n903 = local read "RESET"() -> (w1046:bool)
          n904 = property on="balanza2" class="Bool (strict)"() -> ("Left"=w1050:i32)  [unwired: 2 in, 2 out]
          n905 = Less?(x=w1050, y=965) -> (x < y?=w1047:bool)
          n906 = Or(x=w1047, y=w1046) -> (x .or. y?=w1048:bool)
        }
        n907 = local write "M19"(FALSE ("M20")) -> ()
        n908 = local write "ANALIZANDO\nCC"(FALSE ("ANALIZANDO\nCC")) -> ()
        n909 = local write "M20"(TRUE ("M21")) -> ()
        n910 = local write "ROJO"(TRUE ("ROJO")) -> ()
        n911 = local write "PESO\nSI"(TRUE ("PESO\nSI")) -> ()
      }
    }
    n912 = case shown="True" w228 {
      frame False {
      }
      frame True {
        n913 = property on="TAPA NEUTRO" class="Bool (strict)"("Visible"=FALSE) -> ()  [unwired: 2 in, 2 out]
        n914 = property on="TAPA AZUL" class="Bool (strict)"("Visible"=TRUE) -> ()  [unwired: 2 in, 2 out]
        n915 = property on="TAPA AZUL" class="Bool (strict)"("Top"=14 ("Position:Top")) -> ()  [unwired: 2 in, 2 out]
        n916 = property on="TAPA AZUL" class="Bool (strict)"("Left"=917 ("Position:Left")) -> ()  [unwired: 2 in, 2 out]
        n917 = property on="MODULO6" class="Bool (strict)"("Left"=378 ("Position:Left")) -> ()  [unwired: 2 in, 2 out]
        n918 = property on="VASTAGO MODULO6" class="Bool (strict)"("Top"=-11 ("Position:Top")) -> ()  [unwired: 2 in, 2 out]
        n919 = property on="CILINDRO MODULO6" class="Bool (strict)"("Left"=376 ("Position:Left")) -> ()  [unwired: 2 in, 2 out]
        n920 = property on="VASTAGO MODULO6" class="Bool (strict)"("Left"=385 ("Position:Left")) -> ()  [unwired: 2 in, 2 out]
        n921 = while {
          stop <- w952 stop-if-true
          n922 = property on="balanza2" class="Bool (strict)"() -> ("Left"=w958:i32)  [unwired: 2 in, 2 out]
          n923 = Subtract(x=w958, y=3) -> (x-y=w959:i32)
          n924 = property on="balanza2" class="Bool (strict)"("Left"=w959) -> ()  [unwired: 2 in, 2 out]
          n925 = Wait (ms)(milliseconds to wait=u32 0) -> ()  [unwired: 1 out]
          n926 = local read "RESET"() -> (w951:bool)
          n927 = property on="balanza2" class="Bool (strict)"() -> ("Left"=w955:i32)  [unwired: 2 in, 2 out]
          n928 = Less?(x=w955, y=965) -> (x < y?=w953:bool)
          n929 = Or(x=w953, y=w951) -> (x .or. y?=w952:bool)
        }
        n930 = local write "M19"(FALSE ("M19")) -> ()
        n931 = local write "ANALIZANDO\nCC"(FALSE ("ANALIZANDO\nCC")) -> ()
        n932 = local write "AZUL"(TRUE ("AZUL")) -> ()
        n933 = local write "PESO\nSI"(TRUE ("PESO\nSI")) -> ()
        n934 = local write "M26"(TRUE ("M26")) -> ()
      }
    }
    n935 = case shown="True" w208 {
      frame False {
      }
      frame True {
        n936 = while {
          stop <- w881 stop-if-true
          n937 = property on="TAPA AZUL" class="Bool (strict)"() -> ("Left"=w898:i32)  [unwired: 2 in, 2 out]
          n938 = Subtract(x=w898, y=2) -> (x-y=w896:i32)
          n939 = property on="TAPA AZUL" class="Bool (strict)"("Left"=w896) -> ()  [unwired: 2 in, 2 out]
          n940 = property on="CILINDRO MODULO6" class="Bool (strict)"() -> ("Left"=w895:i32)  [unwired: 2 in, 2 out]
          n941 = Subtract(x=w895, y=2) -> (x-y=w893:i32)
          n942 = property on="CILINDRO MODULO6" class="Bool (strict)"("Left"=w893) -> ()  [unwired: 2 in, 2 out]
          n943 = property on="VASTAGO MODULO6" class="Bool (strict)"() -> ("Left"=w892:i32)  [unwired: 2 in, 2 out]
          n944 = Subtract(x=w892, y=2) -> (x-y=w890:i32)
          n945 = property on="VASTAGO MODULO6" class="Bool (strict)"("Left"=w890) -> ()  [unwired: 2 in, 2 out]
          n946 = property on="MODULO6" class="Bool (strict)"() -> ("Left"=w889:i32)  [unwired: 2 in, 2 out]
          n947 = Subtract(x=w889, y=2) -> (x-y=w887:i32)
          n948 = property on="MODULO6" class="Bool (strict)"("Left"=w887) -> ()  [unwired: 2 in, 2 out]
          n949 = Wait (ms)(milliseconds to wait=u32 0) -> ()  [unwired: 1 out]
          n950 = local read "RESET"() -> (w883:bool)
          n951 = property on="MODULO6" class="Bool (strict)"() -> ("Left"=w886:i32)  [unwired: 2 in, 2 out]
          n952 = Less?(x=w886, y=316) -> (x < y?=w884:bool)
          n953 = Or(x=w884, y=w883) -> (x .or. y?=w881:bool)
        }
        n954 = local write "M29"(FALSE ("M29")) -> ()
        n955 = local write "M30"(TRUE ("M30")) -> ()
      }
    }
    n956 = case shown="True" w193 {
      frame False {
      }
      frame True {
        n957 = while {
          stop <- w835 stop-if-true
          n958 = property on="CILINDRO MODULO6" class="Bool (strict)"() -> ("Left"=w849:i32)  [unwired: 2 in, 2 out]
          n959 = Add(x=w849, y=3) -> (x+y=w847:i32)
          n960 = property on="CILINDRO MODULO6" class="Bool (strict)"("Left"=w847) -> ()  [unwired: 2 in, 2 out]
          n961 = property on="VASTAGO MODULO6" class="Bool (strict)"() -> ("Left"=w846:i32)  [unwired: 2 in, 2 out]
          n962 = Add(x=w846, y=3) -> (x+y=w844:i32)
          n963 = property on="VASTAGO MODULO6" class="Bool (strict)"("Left"=w844) -> ()  [unwired: 2 in, 2 out]
          n964 = property on="MODULO6" class="Bool (strict)"() -> ("Left"=w843:i32)  [unwired: 2 in, 2 out]
          n965 = Add(x=w843, y=3) -> (x+y=w841:i32)
          n966 = property on="MODULO6" class="Bool (strict)"("Left"=w841) -> ()  [unwired: 2 in, 2 out]
          n967 = Wait (ms)(milliseconds to wait=u32 0) -> ()  [unwired: 1 out]
          n968 = local read "RESET"() -> (w836:bool)
          n969 = property on="MODULO6" class="Bool (strict)"() -> ("Left"=w839:i32)  [unwired: 2 in, 2 out]
          n970 = Greater?(x=w839, y=377) -> (0:w837:bool)
          n971 = Or(x=w837, y=w836) -> (x .or. y?=w835:bool)
        }
        n972 = local write "M32"(FALSE ("M32")) -> ()
        n973 = local write "M33"(TRUE ("M33")) -> ()
      }
    }
    n974 = case shown="True" w157 {
      frame False {
      }
      frame True {
        n975 = while {
          stop <- w714 stop-if-true
          n976 = property on="VASTAGO RECHAZO" class="Bool (strict)"() -> ("Top"=w728:i32)  [unwired: 2 in, 2 out]
          n977 = Add(x=w728, y=6) -> (x+y=w726:i32)
          n978 = property on="VASTAGO RECHAZO" class="Bool (strict)"("Top"=w726) -> ()  [unwired: 2 in, 2 out]
          n979 = property on="PINZA ABIERTA" class="Bool (strict)"() -> ("Top"=w725:i32)  [unwired: 2 in, 2 out]
          n980 = Add(x=w725, y=6) -> (x+y=w723:i32)
          n981 = property on="PINZA ABIERTA" class="Bool (strict)"("Top"=w723) -> ()  [unwired: 2 in, 2 out]
          n982 = property on="PINZA CERRADA" class="Bool (strict)"() -> ("Top"=w722:i32)  [unwired: 2 in, 2 out]
          n983 = Add(x=w722, y=6) -> (x+y=w720:i32)
          n984 = property on="PINZA CERRADA" class="Bool (strict)"("Top"=w720) -> ()  [unwired: 2 in, 2 out]
          n985 = Wait (ms)(milliseconds to wait=u32 0) -> ()  [unwired: 1 out]
          n986 = local read "RESET"() -> (w715:bool)
          n987 = property on="PINZA CERRADA" class="Bool (strict)"() -> ("Top"=w718:i32)  [unwired: 2 in, 2 out]
          n988 = Greater?(x=w718, y=396) -> (0:w716:bool)
          n989 = Or(x=w716, y=w715) -> (x .or. y?=w714:bool)
        }
        n990 = local write "M38"(FALSE ("M38")) -> ()
        n991 = local write "M39"(TRUE ("M39")) -> ()
      }
    }
    n992 = case shown="True" w142 {
      frame False {
      }
      frame True {
        n993 = while {
          stop <- w641 stop-if-true
          n994 = property on="PINZA ABIERTA" class="Bool (strict)"() -> ("Top"=w658:i32)  [unwired: 2 in, 2 out]
          n995 = Add(x=w658, y=6) -> (x+y=w656:i32)
          n996 = property on="PINZA ABIERTA" class="Bool (strict)"("Top"=w656) -> ()  [unwired: 2 in, 2 out]
          n997 = property on="VASTAGO RECHAZO" class="Bool (strict)"() -> ("Top"=w655:i32)  [unwired: 2 in, 2 out]
          n998 = Add(x=w655, y=6) -> (x+y=w653:i32)
          n999 = property on="VASTAGO RECHAZO" class="Bool (strict)"("Top"=w653) -> ()  [unwired: 2 in, 2 out]
          n1000 = property on="TARRO NOCOLOR" class="Bool (strict)"() -> ("Top"=w652:i32)  [unwired: 2 in, 2 out]
          n1001 = Add(x=w652, y=6) -> (x+y=w650:i32)
          n1002 = property on="TARRO NOCOLOR" class="Bool (strict)"("Top"=w650) -> ()  [unwired: 2 in, 2 out]
          n1003 = property on="PINZA CERRADA" class="Bool (strict)"() -> ("Top"=w649:i32)  [unwired: 2 in, 2 out]
          n1004 = Add(x=w649, y=6) -> (x+y=w647:i32)
          n1005 = property on="PINZA CERRADA" class="Bool (strict)"("Top"=w647) -> ()  [unwired: 2 in, 2 out]
          n1006 = Wait (ms)(milliseconds to wait=u32 0) -> ()  [unwired: 1 out]
          n1007 = local read "RESET"() -> (w642:bool)
          n1008 = property on="PINZA CERRADA" class="Bool (strict)"() -> ("Top"=w645:i32)  [unwired: 2 in, 2 out]
          n1009 = Greater?(x=w645, y=396) -> (0:w643:bool)
          n1010 = Or(x=w643, y=w642) -> (x .or. y?=w641:bool)
        }
        n1011 = local write "M41"(FALSE ("M41")) -> ()
        n1012 = local write "M42"(TRUE ("M42")) -> ()
      }
    }
    n1013 = case shown="True" w100 {
      frame False {
      }
      frame True {
        n1014 = while {
          stop <- w490 stop-if-true
          n1015 = property on="VASTAGO RECHAZO" class="Bool (strict)"() -> ("Top"=w504:i32)  [unwired: 2 in, 2 out]
          n1016 = Add(x=w504, y=6) -> (x+y=w502:i32)
          n1017 = property on="VASTAGO RECHAZO" class="Bool (strict)"("Top"=w502) -> ()  [unwired: 2 in, 2 out]
          n1018 = property on="PINZA ABIERTA" class="Bool (strict)"() -> ("Top"=w501:i32)  [unwired: 2 in, 2 out]
          n1019 = Add(x=w501, y=6) -> (x+y=w499:i32)
          n1020 = property on="PINZA ABIERTA" class="Bool (strict)"("Top"=w499) -> ()  [unwired: 2 in, 2 out]
          n1021 = property on="PINZA CERRADA" class="Bool (strict)"() -> ("Top"=w498:i32)  [unwired: 2 in, 2 out]
          n1022 = Add(x=w498, y=6) -> (x+y=w496:i32)
          n1023 = property on="PINZA CERRADA" class="Bool (strict)"("Top"=w496) -> ()  [unwired: 2 in, 2 out]
          n1024 = Wait (ms)(milliseconds to wait=u32 0) -> ()  [unwired: 1 out]
          n1025 = local read "RESET"() -> (w491:bool)
          n1026 = property on="PINZA CERRADA" class="Bool (strict)"() -> ("Top"=w494:i32)  [unwired: 2 in, 2 out]
          n1027 = Greater?(x=w494, y=396) -> (0:w492:bool)
          n1028 = Or(x=w492, y=w491) -> (x .or. y?=w490:bool)
        }
        n1029 = local write "M48"(FALSE ("M48")) -> ()
        n1030 = local write "M49"(TRUE ("M49")) -> ()
      }
    }
    n1031 = case shown="True" w85 {
      frame False {
      }
      frame True {
        n1032 = while {
          stop <- w416 stop-if-true
          n1033 = property on="PINZA ABIERTA" class="Bool (strict)"() -> ("Top"=w433:i32)  [unwired: 2 in, 2 out]
          n1034 = Add(x=w433, y=6) -> (x+y=w431:i32)
          n1035 = property on="PINZA ABIERTA" class="Bool (strict)"("Top"=w431) -> ()  [unwired: 2 in, 2 out]
          n1036 = property on="VASTAGO RECHAZO" class="Bool (strict)"() -> ("Top"=w430:i32)  [unwired: 2 in, 2 out]
          n1037 = Add(x=w430, y=6) -> (x+y=w428:i32)
          n1038 = property on="VASTAGO RECHAZO" class="Bool (strict)"("Top"=w428) -> ()  [unwired: 2 in, 2 out]
          n1039 = property on="TARRO NOPESO" class="Bool (strict)"() -> ("Top"=w427:i32)  [unwired: 2 in, 2 out]
          n1040 = Add(x=w427, y=6) -> (x+y=w425:i32)
          n1041 = property on="TARRO NOPESO" class="Bool (strict)"("Top"=w425) -> ()  [unwired: 2 in, 2 out]
          n1042 = property on="PINZA CERRADA" class="Bool (strict)"() -> ("Top"=w424:i32)  [unwired: 2 in, 2 out]
          n1043 = Add(x=w424, y=6) -> (x+y=w422:i32)
          n1044 = property on="PINZA CERRADA" class="Bool (strict)"("Top"=w422) -> ()  [unwired: 2 in, 2 out]
          n1045 = Wait (ms)(milliseconds to wait=u32 0) -> ()  [unwired: 1 out]
          n1046 = local read "RESET"() -> (w417:bool)
          n1047 = property on="PINZA CERRADA" class="Bool (strict)"() -> ("Top"=w420:i32)  [unwired: 2 in, 2 out]
          n1048 = Greater?(x=w420, y=396) -> (0:w418:bool)
          n1049 = Or(x=w418, y=w417) -> (x .or. y?=w416:bool)
        }
        n1050 = local write "M51"(FALSE ("M51")) -> ()
        n1051 = local write "M52"(TRUE ("M52")) -> ()
      }
    }
    n1052 = case shown="True" w298 {
      frame False {
      }
      frame True {
        n1053 = property on="CAJA LLENA" class="Bool (strict)"("Visible"=FALSE) -> ()  [unwired: 2 in, 2 out]
        n1054 = while {
          stop <- w1146 stop-if-true
          n1055 = property on="CILINDRO NUEVO" class="Bool (strict)"() -> ("Left"=w1162:i32)  [unwired: 2 in, 2 out]
          n1056 = Subtract(x=w1162, y=1) -> (x-y=w1160:i32)
          n1057 = property on="CILINDRO NUEVO" class="Bool (strict)"("Left"=w1160) -> ()  [unwired: 2 in, 2 out]
          n1058 = property on="BASTAGO TAPAS" class="Bool (strict)"() -> ("Left"=w1157:i32)  [unwired: 2 in, 2 out]
          n1059 = Add(x=w1157, y=3) -> (x+y=w1155:i32)
          n1060 = property on="BASTAGO TAPAS" class="Bool (strict)"("Left"=w1155) -> ()  [unwired: 2 in, 2 out]
          n1061 = property on="vastago1 tapado" class="Bool (strict)"() -> ("Left"=w1153:i32)  [unwired: 2 in, 2 out]
          n1062 = Subtract(x=w1153, y=3) -> (x-y=w1151:i32)
          n1063 = property on="vastago1 tapado" class="Bool (strict)"("Left"=w1151) -> ()  [unwired: 2 in, 2 out]
          n1064 = property on="vastago2 tapado" class="Bool (strict)"() -> ("Left"=w1150:i32)  [unwired: 2 in, 2 out]
          n1065 = Add(x=w1150, y=1) -> (x+y=w1148:i32)
          n1066 = property on="vastago2 tapado" class="Bool (strict)"("Left"=w1148) -> ()  [unwired: 2 in, 2 out]
          n1067 = Wait (ms)(milliseconds to wait=u32 0) -> ()  [unwired: 1 out]
          n1068 = local read "RESET"() -> (w1145:bool)
          n1069 = property on="CILINDRO NUEVO" class="Bool (strict)"() -> ("Left"=w1159:i32)  [unwired: 2 in, 2 out]
          n1070 = Less?(x=w1159, y=870) -> (x < y?=w1154:bool)
          n1071 = Or(x=w1154, y=w1145) -> (x .or. y?=w1146:bool)
        }
        n1072 = local write "M12"(FALSE ("M12")) -> ()
        n1073 = local write "M13"(TRUE ("M13")) -> ()
      }
    }
    n1074 = case shown="True" w152 {
      frame False {
      }
      frame True {
        n1075 = property on="PINZA CERRADA" class="Bool (strict)"("Visible"=TRUE) -> ()  [unwired: 2 in, 2 out]
        n1076 = property on="PINZA ABIERTA" class="Bool (strict)"("Visible"=FALSE) -> ()  [unwired: 2 in, 2 out]
        n1077 = while {
          stop <- w695 stop-if-true
          n1078 = property on="PINZA ABIERTA" class="Bool (strict)"() -> ("Top"=w711:i32)  [unwired: 2 in, 2 out]
          n1079 = Subtract(x=w711, y=6) -> (x-y=w709:i32)
          n1080 = property on="PINZA ABIERTA" class="Bool (strict)"("Top"=w709) -> ()  [unwired: 2 in, 2 out]
          n1081 = property on="VASTAGO RECHAZO" class="Bool (strict)"() -> ("Top"=w708:i32)  [unwired: 2 in, 2 out]
          n1082 = Subtract(x=w708, y=6) -> (x-y=w706:i32)
          n1083 = property on="VASTAGO RECHAZO" class="Bool (strict)"("Top"=w706) -> ()  [unwired: 2 in, 2 out]
          n1084 = property on="TARRO NOCOLOR" class="Bool (strict)"() -> ("Top"=w705:i32)  [unwired: 2 in, 2 out]
          n1085 = Subtract(x=w705, y=6) -> (x-y=w703:i32)
          n1086 = property on="TARRO NOCOLOR" class="Bool (strict)"("Top"=w703) -> ()  [unwired: 2 in, 2 out]
          n1087 = property on="PINZA CERRADA" class="Bool (strict)"() -> ("Top"=w702:i32)  [unwired: 2 in, 2 out]
          n1088 = Subtract(x=w702, y=6) -> (x-y=w700:i32)
          n1089 = property on="PINZA CERRADA" class="Bool (strict)"("Top"=w700) -> ()  [unwired: 2 in, 2 out]
          n1090 = local read "RESET"() -> (w696:bool)
          n1091 = property on="PINZA CERRADA" class="Bool (strict)"() -> ("Top"=w699:i32)  [unwired: 2 in, 2 out]
          n1092 = Less?(x=w699, y=317) -> (x < y?=w697:bool)
          n1093 = Or(x=w697, y=w696) -> (x .or. y?=w695:bool)
        }
        n1094 = local write "M40"(TRUE ("M40")) -> ()
        n1095 = local write "M39"(FALSE ("M39")) -> ()
      }
    }
    n1096 = case shown="True" w127 {
      frame False {
      }
      frame True {
        n1097 = property on="TAPA NEUTRO" class="Bool (strict)"("Visible"=FALSE) -> ()  [unwired: 2 in, 2 out]
        n1098 = property on="TAPA NOPESO" class="Bool (strict)"("Visible"=TRUE) -> ()  [unwired: 2 in, 2 out]
        n1099 = property on="ACTUADOR RECHAZO" class="Bool (strict)"("Top"=220 ("Position:Top")) -> ()  [unwired: 2 in, 2 out]
        n1100 = property on="CILINDRO RECHAZO" class="Bool (strict)"("Left"=592 ("Position:Left")) -> ()  [unwired: 2 in, 2 out]
        n1101 = property on="VASTAGO RECHAZO" class="Bool (strict)"("Top"=180 ("Position:Top")) -> ()  [unwired: 2 in, 2 out]
        n1102 = property on="CILINDRO RECHAZO1" class="Bool (strict)"("Left"=620 ("Position:Left")) -> ()  [unwired: 2 in, 2 out]
        n1103 = property on="VASTAGO RECHAZO" class="Bool (strict)"("Left"=614 ("Position:Left")) -> ()  [unwired: 2 in, 2 out]
        n1104 = property on="TAPA NOPESO" class="Bool (strict)"("Left"=917 ("Position:Left")) -> ()  [unwired: 2 in, 2 out]
        n1105 = property on="TAPA NOPESO" class="Bool (strict)"("Top"=14 ("Position:Top")) -> ()  [unwired: 2 in, 2 out]
        n1106 = property on="PINZA CERRADA" class="Bool (strict)"("Left"=596 ("Position:Left")) -> ()  [unwired: 2 in, 2 out]
        n1107 = property on="PINZA CERRADA" class="Bool (strict)"("Top"=316 ("Position:Top")) -> ()  [unwired: 2 in, 2 out]
        n1108 = property on="PINZA ABIERTA" class="Bool (strict)"("Left"=587 ("Position:Left")) -> ()  [unwired: 2 in, 2 out]
        n1109 = property on="PINZA ABIERTA" class="Bool (strict)"("Top"=313 ("Position:Top")) -> ()  [unwired: 2 in, 2 out]
        n1110 = property on="TARRO NOPESO" class="Bool (strict)"("Left"=386 ("Position:Left")) -> ()  [unwired: 2 in, 2 out]
        n1111 = property on="TARRO NOPESO" class="Bool (strict)"("Top"=409 ("Position:Top")) -> ()  [unwired: 2 in, 2 out]
        n1112 = while {
          stop <- w597 stop-if-true
          n1113 = property on="balanza2" class="Bool (strict)"() -> ("Left"=w605:i32)  [unwired: 2 in, 2 out]
          n1114 = Subtract(x=w605, y=6) -> (x-y=w603:i32)
          n1115 = property on="balanza2" class="Bool (strict)"("Left"=w603) -> ()  [unwired: 2 in, 2 out]
          n1116 = Wait (ms)(milliseconds to wait=u32 0) -> ()  [unwired: 1 out]
          n1117 = local read "RESET"() -> (w598:bool)
          n1118 = property on="balanza2" class="Bool (strict)"() -> ("Left"=w602:i32)  [unwired: 2 in, 2 out]
          n1119 = Less?(x=w602, y=965) -> (x < y?=w599:bool)
          n1120 = Or(x=w599, y=w598) -> (x .or. y?=w597:bool)
        }
        n1121 = local write "ANALIZANDO\nCC"(FALSE ("ANALIZANDO\nCC")) -> ()
        n1122 = local write "PESO\nNO"(TRUE ("PESO\nNO")) -> ()
        n1123 = local write "M19"(FALSE ("M19")) -> ()
        n1124 = local write "M44"(TRUE ("M44")) -> ()
      }
    }
    n1125 = case shown="True" w95 {
      frame False {
      }
      frame True {
        n1126 = property on="PINZA ABIERTA" class="Bool (strict)"("Visible"=FALSE) -> ()  [unwired: 2 in, 2 out]
        n1127 = property on="PINZA CERRADA" class="Bool (strict)"("Visible"=TRUE) -> ()  [unwired: 2 in, 2 out]
        n1128 = while {
          stop <- w470 stop-if-true
          n1129 = property on="PINZA ABIERTA" class="Bool (strict)"() -> ("Top"=w487:i32)  [unwired: 2 in, 2 out]
          n1130 = Subtract(x=w487, y=6) -> (x-y=w485:i32)
          n1131 = property on="PINZA ABIERTA" class="Bool (strict)"("Top"=w485) -> ()  [unwired: 2 in, 2 out]
          n1132 = property on="VASTAGO RECHAZO" class="Bool (strict)"() -> ("Top"=w484:i32)  [unwired: 2 in, 2 out]
          n1133 = Subtract(x=w484, y=6) -> (x-y=w482:i32)
          n1134 = property on="VASTAGO RECHAZO" class="Bool (strict)"("Top"=w482) -> ()  [unwired: 2 in, 2 out]
          n1135 = property on="TARRO NOPESO" class="Bool (strict)"() -> ("Top"=w481:i32)  [unwired: 2 in, 2 out]
          n1136 = Subtract(x=w481, y=6) -> (x-y=w479:i32)
          n1137 = property on="TARRO NOPESO" class="Bool (strict)"("Top"=w479) -> ()  [unwired: 2 in, 2 out]
          n1138 = property on="PINZA CERRADA" class="Bool (strict)"() -> ("Top"=w478:i32)  [unwired: 2 in, 2 out]
          n1139 = Subtract(x=w478, y=6) -> (x-y=w476:i32)
          n1140 = property on="PINZA CERRADA" class="Bool (strict)"("Top"=w476) -> ()  [unwired: 2 in, 2 out]
          n1141 = Wait (ms)(milliseconds to wait=u32 0) -> ()  [unwired: 1 out]
          n1142 = local read "RESET"() -> (w471:bool)
          n1143 = property on="PINZA CERRADA" class="Bool (strict)"() -> ("Top"=w474:i32)  [unwired: 2 in, 2 out]
          n1144 = Less?(x=w474, y=317) -> (x < y?=w472:bool)
          n1145 = Or(x=w472, y=w471) -> (x .or. y?=w470:bool)
        }
        n1146 = local write "M49"(FALSE ("M49")) -> ()
        n1147 = local write "M50"(TRUE ("M50")) -> ()
      }
    }
    n1148 = case shown="True" w62 {
      frame False {
      }
      frame True {
        n1149 = property on="TARRO VACIO" class="Bool (strict)"("Top"=412 ("Position:Top")) -> ()  [unwired: 2 in, 2 out]
        n1150 = property on="PUERTA TOLVA" class="Bool (strict)"("Left"=929 ("Position:Left")) -> ()  [unwired: 2 in, 2 out]
        n1151 = property on="CAJA LLENA" class="Bool (strict)"("Top"=250 ("Position:Top")) -> ()  [unwired: 2 in, 2 out]
        n1152 = property on="BALANZA1" class="Bool (strict)"("Top"=146 ("Position:Top")) -> ()  [unwired: 2 in, 2 out]
        n1153 = property on="CILINDRO NUEVO" class="Bool (strict)"("Left"=869 ("Position:Left")) -> ()  [unwired: 2 in, 2 out]
        n1154 = property on="TAPA NEUTRO" class="Bool (strict)"("Left"=980 ("Position:Left")) -> ()  [unwired: 2 in, 2 out]
        n1155 = property on="TAPA NEUTRO" class="Bool (strict)"("Top"=96 ("Position:Top")) -> ()  [unwired: 2 in, 2 out]
        n1156 = property on="TARRO VACIO" class="Bool (strict)"("Visible"=FALSE) -> ()  [unwired: 2 in, 2 out]
        n1157 = property on="TAPA NEUTRO" class="Bool (strict)"("Visible"=FALSE) -> ()  [unwired: 2 in, 2 out]
        n1158 = property on="TARRO NOPESO" class="Bool (strict)"("Visible"=FALSE) -> ()  [unwired: 2 in, 2 out]
        n1159 = property on="estructura1" class="Bool (strict)"("Visible"=FALSE) -> ()  [unwired: 2 in, 2 out]
        n1160 = property on="TAPA NOPESO" class="Bool (strict)"("Visible"=FALSE) -> ()  [unwired: 2 in, 2 out]
        n1161 = property on="tarro vaciop" class="Bool (strict)"("Visible"=FALSE) -> ()  [unwired: 2 in, 2 out]
        n1162 = property on="vastagoaux1" class="Bool (strict)"("Visible"=FALSE) -> ()  [unwired: 2 in, 2 out]
        n1163 = property on="cuadroblanco" class="Bool (strict)"("Visible"=FALSE) -> ()  [unwired: 2 in, 2 out]
        n1164 = property on="TAPA TARRO ROJO" class="Bool (strict)"("Visible"=FALSE) -> ()  [unwired: 2 in, 2 out]
        n1165 = property on="VASTAGO MODULO6" class="Bool (strict)"("Top"=-11 ("Position:Top")) -> ()  [unwired: 2 in, 2 out]
        n1166 = property on="VASTAGO MODULO6" class="Bool (strict)"("Left"=385 ("Position:Left")) -> ()  [unwired: 2 in, 2 out]
        n1167 = property on="TAPA AZUL" class="Bool (strict)"("Left"=917 ("Position:Left")) -> ()  [unwired: 2 in, 2 out]
        n1168 = property on="MODULO6" class="Bool (strict)"("Left"=378 ("Position:Left")) -> ()  [unwired: 2 in, 2 out]
        n1169 = property on="CILINDRO MODULO6" class="Bool (strict)"("Left"=376 ("Position:Left")) -> ()  [unwired: 2 in, 2 out]
        n1170 = property on="TAPA AZUL" class="Bool (strict)"("Top"=14 ("Position:Top")) -> ()  [unwired: 2 in, 2 out]
        n1171 = property on="TAPA AZUL" class="Bool (strict)"("Visible"=FALSE) -> ()  [unwired: 2 in, 2 out]
        n1172 = property on="CAJA LLENA" class="Bool (strict)"("Visible"=FALSE) -> ()  [unwired: 2 in, 2 out]
        n1173 = property on="dep inferior" class="Bool (strict)"("Visible"=FALSE) -> ()  [unwired: 2 in, 2 out]
        n1174 = property on="dep superior" class="Bool (strict)"("Visible"=FALSE) -> ()  [unwired: 2 in, 2 out]
        n1175 = property on="cilindros tolva" class="Bool (strict)"("Visible"=FALSE) -> ()  [unwired: 2 in, 2 out]
        n1176 = property on="puerta tolva2" class="Bool (strict)"("Visible"=FALSE) -> ()  [unwired: 2 in, 2 out]
        n1177 = property on="perta tolva1" class="Bool (strict)"("Visible"=FALSE) -> ()  [unwired: 2 in, 2 out]
        n1178 = property on="BASTAGO TAPAS" class="Bool (strict)"("Left"=973 ("Position:Left")) -> ()  [unwired: 2 in, 2 out]
        n1179 = property on="vastagoaux1" class="Bool (strict)"("Top"=420 ("Position:Top")) -> ()  [unwired: 2 in, 2 out]
        n1180 = property on="tarro vaciop" class="Bool (strict)"("Top"=358 ("Position:Top")) -> ()  [unwired: 2 in, 2 out]
        n1181 = property on="tapa neutrop" class="Bool (strict)"("Left"=527 ("Position:Left")) -> ()  [unwired: 2 in, 2 out]
        n1182 = property on="tapa neutrop" class="Bool (strict)"("Top"=345 ("Position:Top")) -> ()  [unwired: 2 in, 2 out]
        n1183 = property on="vastago1 tapado" class="Bool (strict)"("Left"=361 ("Position:Left")) -> ()  [unwired: 2 in, 2 out]
        n1184 = property on="balanza2" class="Bool (strict)"("Left"=978 ("Position:Left")) -> ()  [unwired: 2 in, 2 out]
        n1185 = property on="PINZA ABIERTA" class="Bool (strict)"("Visible"=FALSE) -> ()  [unwired: 2 in, 2 out]
        n1186 = property on="TAPA NOCOLOR" class="Bool (strict)"("Left"=917 ("Position:Left")) -> ()  [unwired: 2 in, 2 out]
        n1187 = property on="VASTAGO RECHAZO" class="Bool (strict)"("Visible"=FALSE) -> ()  [unwired: 2 in, 2 out]
        n1188 = property on="ACTUADOR RECHAZO" class="Bool (strict)"("Top"=220 ("Position:Top")) -> ()  [unwired: 2 in, 2 out]
        n1189 = property on="TAPA NOCOLOR" class="Bool (strict)"("Top"=14 ("Position:Top")) -> ()  [unwired: 2 in, 2 out]
        n1190 = property on="TARRO NOCOLOR" class="Bool (strict)"("Visible"=FALSE) -> ()  [unwired: 2 in, 2 out]
        n1191 = property on="TARRO NOCOLOR" class="Bool (strict)"("Left"=386 ("Position:Left")) -> ()  [unwired: 2 in, 2 out]
        n1192 = property on="PINZA ABIERTA" class="Bool (strict)"("Top"=313 ("Position:Top")) -> ()  [unwired: 2 in, 2 out]
        n1193 = property on="PINZA ABIERTA" class="Bool (strict)"("Left"=587 ("Position:Left")) -> ()  [unwired: 2 in, 2 out]
        n1194 = property on="tolva vacia" class="Bool (strict)"("Visible"=FALSE) -> ()  [unwired: 2 in, 2 out]
        n1195 = property on="tarro vaciop1" class="Bool (strict)"("Visible"=FALSE) -> ()  [unwired: 2 in, 2 out]
        n1196 = property on="tarro llenop" class="Bool (strict)"("Visible"=FALSE) -> ()  [unwired: 2 in, 2 out]
        n1197 = property on="estructura tapado" class="Bool (strict)"("Visible"=FALSE) -> ()  [unwired: 2 in, 2 out]
        n1198 = property on="tapa neutrop" class="Bool (strict)"("Visible"=FALSE) -> ()  [unwired: 2 in, 2 out]
        n1199 = property on="vastago1 tapado" class="Bool (strict)"("Visible"=FALSE) -> ()  [unwired: 2 in, 2 out]
        n1200 = local write "ROJO"(FALSE ("ROJO")) -> ()
        n1201 = local write "AZUL"(FALSE ("AZUL")) -> ()
        n1202 = local write "PESO\nSI"(FALSE ("PESO\nSI")) -> ()
        n1203 = property on="cilindro1 tapado" class="Bool (strict)"("Visible"=FALSE) -> ()  [unwired: 2 in, 2 out]
        n1204 = property on="vastago2 tapado" class="Bool (strict)"("Visible"=FALSE) -> ()  [unwired: 2 in, 2 out]
        n1205 = property on="CILINDRO RECHAZO1" class="Bool (strict)"("Visible"=FALSE) -> ()  [unwired: 2 in, 2 out]
        n1206 = property on="cilindro2 tapado" class="Bool (strict)"("Visible"=FALSE) -> ()  [unwired: 2 in, 2 out]
        n1207 = property on="TAPA NOCOLOR" class="Bool (strict)"("Visible"=FALSE) -> ()  [unwired: 2 in, 2 out]
        n1208 = property on="CILINDRO RECHAZO" class="Bool (strict)"("Visible"=FALSE) -> ()  [unwired: 2 in, 2 out]
        n1209 = property on="vastago3 tapado" class="Bool (strict)"("Visible"=FALSE) -> ()  [unwired: 2 in, 2 out]
        n1210 = property on="cilindro3 tapado" class="Bool (strict)"("Visible"=FALSE) -> ()  [unwired: 2 in, 2 out]
        n1211 = property on="TARRO NOCOLOR" class="Bool (strict)"("Top"=409 ("Position:Top")) -> ()  [unwired: 2 in, 2 out]
        n1212 = property on="vastago4 tapado" class="Bool (strict)"("Visible"=FALSE) -> ()  [unwired: 2 in, 2 out]
        n1213 = property on="vastago2 tapado" class="Bool (strict)"("Left"=626 ("Position:Left")) -> ()  [unwired: 2 in, 2 out]
        n1214 = property on="vastago3 tapado" class="Bool (strict)"("Top"=206 ("Position:Top")) -> ()  [unwired: 2 in, 2 out]
        n1215 = property on="CILINDRO RECHAZO" class="Bool (strict)"("Left"=592 ("Position:Left")) -> ()  [unwired: 2 in, 2 out]
        n1216 = property on="CILINDRO RECHAZO1" class="Bool (strict)"("Left"=620 ("Position:Left")) -> ()  [unwired: 2 in, 2 out]
        n1217 = property on="vastago4 tapado" class="Bool (strict)"("Top"=226 ("Position:Top")) -> ()  [unwired: 2 in, 2 out]
        n1218 = property on="puerta tolva2" class="Bool (strict)"("Left"=450 ("Position:Left")) -> ()  [unwired: 2 in, 2 out]
        n1219 = property on="perta tolva1" class="Bool (strict)"("Left"=450 ("Position:Left")) -> ()  [unwired: 2 in, 2 out]
        n1220 = property on="VASTAGO RECHAZO" class="Bool (strict)"("Left"=614 ("Position:Left")) -> ()  [unwired: 2 in, 2 out]
        n1221 = property on="TAPA TARRO ROJO" class="Bool (strict)"("Left"=916 ("Position:Left")) -> ()  [unwired: 2 in, 2 out]
        n1222 = property on="TAPA TARRO ROJO" class="Bool (strict)"("Top"=14 ("Position:Top")) -> ()  [unwired: 2 in, 2 out]
        n1223 = local write "ANALIZANDO\nCC"(FALSE ("ANALIZANDO\nCC")) -> ()
        n1224 = local write "PESO\nNO"(FALSE ("PESO\nNO")) -> ()
        n1225 = local write "NO \nCOLOR"(FALSE ("NO \nCOLOR")) -> ()
        n1226 = property on="PINZA CERRADA" class="Bool (strict)"("Visible"=FALSE) -> ()  [unwired: 2 in, 2 out]
        n1227 = property on="ESTRUCTURA RECHAZO" class="Bool (strict)"("Visible"=FALSE) -> ()  [unwired: 2 in, 2 out]
        n1228 = property on="PINZA CERRADA" class="Bool (strict)"("Left"=596 ("Position:Left")) -> ()  [unwired: 2 in, 2 out]
        n1229 = property on="PINZA CERRADA" class="Bool (strict)"("Top"=316 ("Position:Top")) -> ()  [unwired: 2 in, 2 out]
        n1230 = property on="TAPA NOPESO" class="Bool (strict)"("Top"=14 ("Position:Top")) -> ()  [unwired: 2 in, 2 out]
        n1231 = property on="TARRO NOPESO" class="Bool (strict)"("Left"=386 ("Position:Left")) -> ()  [unwired: 2 in, 2 out]
        n1232 = property on="TARRO NOPESO" class="Bool (strict)"("Top"=409 ("Position:Top")) -> ()  [unwired: 2 in, 2 out]
        n1233 = property on="TAPA NOPESO" class="Bool (strict)"("Left"=917 ("Position:Left")) -> ()  [unwired: 2 in, 2 out]
        n1234 = property on="VASTAGO RECHAZO" class="Bool (strict)"("Top"=180 ("Position:Top")) -> ()  [unwired: 2 in, 2 out]
        n1235 = local write "M19"(FALSE ("M19")) -> ()
        n1236 = local write "M12"(FALSE ("M12")) -> ()
        n1237 = local write "M13"(FALSE ("M13")) -> ()
        n1238 = local write "M14"(FALSE ("M14")) -> ()
        n1239 = local write "M15"(FALSE ("M15")) -> ()
        n1240 = local write "M16"(FALSE ("M16")) -> ()
        n1241 = local write "M17"(FALSE ("M17")) -> ()
        n1242 = local write "M18"(FALSE ("M18")) -> ()
        n1243 = local write "M10"(FALSE ("M10")) -> ()
        n1244 = local write "M11"(FALSE ("M11")) -> ()
        n1245 = local write "M9"(FALSE ("M9")) -> ()
        n1246 = local write "M6"(FALSE ("M6")) -> ()
        n1247 = local write "M7"(FALSE ("M7")) -> ()
        n1248 = local write "M8"(FALSE ("M8")) -> ()
        n1249 = local write "M3"(FALSE ("M3")) -> ()
        n1250 = local write "M4"(FALSE ("M4")) -> ()
        n1251 = local write "M5"(FALSE ("M5")) -> ()
        n1252 = local write "M2"(FALSE ("M2")) -> ()
        n1253 = local write "M1"(FALSE ("M1")) -> ()
        n1254 = property on="DEPOSITO NOPESO" class="Bool (strict)"("Visible"=FALSE) -> ()  [unwired: 2 in, 2 out]
        n1255 = property on="DEPOSITO NOCOLOR" class="Bool (strict)"("Visible"=FALSE) -> ()  [unwired: 2 in, 2 out]
        n1256 = local write "M27"(FALSE ("M27")) -> ()
        n1257 = local write "M34"(FALSE ("M34")) -> ()
        n1258 = local write "M26"(FALSE ("M26")) -> ()
        n1259 = local write "M30"(FALSE ("M30")) -> ()
        n1260 = local write "M31"(FALSE ("M31")) -> ()
        n1261 = local write "M32"(FALSE ("M32")) -> ()
        n1262 = local write "M33"(FALSE ("M33")) -> ()
        n1263 = local write "M24"(FALSE ("M24")) -> ()
        n1264 = local write "M25"(FALSE ("M25")) -> ()
        n1265 = local write "M28"(FALSE ("M28")) -> ()
        n1266 = local write "M29"(FALSE ("M29")) -> ()
        n1267 = local write "M21"(FALSE ("M21")) -> ()
        n1268 = local write "M23"(FALSE ("M23")) -> ()
        n1269 = local write "M35"(FALSE ("M35")) -> ()
        n1270 = local write "M20"(FALSE ("M20")) -> ()
        n1271 = local write "M22"(FALSE ("M22")) -> ()
        n1272 = local write "M36"(FALSE ("M36")) -> ()
        n1273 = local write "M54"(FALSE ("M54")) -> ()
        n1274 = local write "M43"(FALSE ("M43")) -> ()
        n1275 = local write "M44"(FALSE ("M44")) -> ()
        n1276 = local write "M51"(FALSE ("M51")) -> ()
        n1277 = local write "M52"(FALSE ("M52")) -> ()
        n1278 = local write "M53"(FALSE ("M53")) -> ()
        n1279 = local write "M41"(FALSE ("M41")) -> ()
        n1280 = local write "M42"(FALSE ("M42")) -> ()
        n1281 = local write "M50"(FALSE ("M50")) -> ()
        n1282 = local write "M38"(FALSE ("M38")) -> ()
        n1283 = local write "M39"(FALSE ("M39")) -> ()
        n1284 = local write "M40"(FALSE ("M40")) -> ()
        n1285 = local write "M45"(FALSE ("M45")) -> ()
        n1286 = local write "M49"(FALSE ("M49")) -> ()
        n1287 = local write "M37"(FALSE ("M37")) -> ()
        n1288 = local write "M46"(FALSE ("M46")) -> ()
        n1289 = local write "M48"(FALSE ("M48")) -> ()
        n1290 = local write "M47"(FALSE ("M47")) -> ()
      }
    }
    n1291 = case shown="True" w137 {
      frame False {
      }
      frame True {
        n1292 = property on="PINZA CERRADA" class="Bool (strict)"("Visible"=FALSE) -> ()  [unwired: 2 in, 2 out]
        n1293 = property on="PINZA ABIERTA" class="Bool (strict)"("Visible"=TRUE) -> ()  [unwired: 2 in, 2 out]
        n1294 = local read "FINALIZADOS\nRECHAZADOS"() -> (w618:dbl)
        n1295 = Increment(x=w618) -> (x+1=w617:dbl)
        n1296 = local write "FINALIZADOS\nRECHAZADOS"(w617) -> ()
        n1297 = while {
          stop <- w624 stop-if-true
          n1298 = property on="PINZA ABIERTA" class="Bool (strict)"() -> ("Top"=w638:i32)  [unwired: 2 in, 2 out]
          n1299 = Subtract(x=w638, y=6) -> (x-y=w636:i32)
          n1300 = property on="PINZA ABIERTA" class="Bool (strict)"("Top"=w636) -> ()  [unwired: 2 in, 2 out]
          n1301 = property on="VASTAGO RECHAZO" class="Bool (strict)"() -> ("Top"=w635:i32)  [unwired: 2 in, 2 out]
          n1302 = Subtract(x=w635, y=6) -> (x-y=w633:i32)
          n1303 = property on="VASTAGO RECHAZO" class="Bool (strict)"("Top"=w633) -> ()  [unwired: 2 in, 2 out]
          n1304 = property on="PINZA CERRADA" class="Bool (strict)"() -> ("Top"=w632:i32)  [unwired: 2 in, 2 out]
          n1305 = Subtract(x=w632, y=6) -> (x-y=w630:i32)
          n1306 = property on="PINZA CERRADA" class="Bool (strict)"("Top"=w630) -> ()  [unwired: 2 in, 2 out]
          n1307 = Wait (ms)(milliseconds to wait=u32 0) -> ()  [unwired: 1 out]
          n1308 = local read "RESET"() -> (w625:bool)
          n1309 = property on="PINZA CERRADA" class="Bool (strict)"() -> ("Top"=w628:i32)  [unwired: 2 in, 2 out]
          n1310 = Less?(x=w628, y=317) -> (x < y?=w626:bool)
          n1311 = Or(x=w626, y=w625) -> (x .or. y?=w624:bool)
        }
        n1312 = local write "M42"(FALSE ("M42")) -> ()
        n1313 = local write "M43"(TRUE ("M43")) -> ()
        n1314 = local write "NO \nCOLOR"(FALSE ("NO \nCOLOR")) -> ()
      }
    }
    n1315 = case shown="True" w80 {
      frame False {
      }
      frame True {
        n1316 = property on="PINZA ABIERTA" class="Bool (strict)"("Visible"=TRUE) -> ()  [unwired: 2 in, 2 out]
        n1317 = property on="PINZA CERRADA" class="Bool (strict)"("Visible"=FALSE) -> ()  [unwired: 2 in, 2 out]
        n1318 = local read "FINALIZADOS\nRECHAZADOS"() -> (w396:dbl)
        n1319 = Increment(x=w396) -> (x+1=w395:dbl)
        n1320 = local write "FINALIZADOS\nRECHAZADOS"(w395) -> ()
        n1321 = while {
          stop <- w399 stop-if-true
          n1322 = property on="PINZA ABIERTA" class="Bool (strict)"() -> ("Top"=w413:i32)  [unwired: 2 in, 2 out]
          n1323 = Subtract(x=w413, y=6) -> (x-y=w411:i32)
          n1324 = property on="PINZA ABIERTA" class="Bool (strict)"("Top"=w411) -> ()  [unwired: 2 in, 2 out]
          n1325 = property on="VASTAGO RECHAZO" class="Bool (strict)"() -> ("Top"=w410:i32)  [unwired: 2 in, 2 out]
          n1326 = Subtract(x=w410, y=6) -> (x-y=w408:i32)
          n1327 = property on="VASTAGO RECHAZO" class="Bool (strict)"("Top"=w408) -> ()  [unwired: 2 in, 2 out]
          n1328 = property on="PINZA CERRADA" class="Bool (strict)"() -> ("Top"=w407:i32)  [unwired: 2 in, 2 out]
          n1329 = Subtract(x=w407, y=6) -> (x-y=w405:i32)
          n1330 = property on="PINZA CERRADA" class="Bool (strict)"("Top"=w405) -> ()  [unwired: 2 in, 2 out]
          n1331 = Wait (ms)(milliseconds to wait=u32 0) -> ()  [unwired: 1 out]
          n1332 = local read "RESET"() -> (w400:bool)
          n1333 = property on="PINZA CERRADA" class="Bool (strict)"() -> ("Top"=w403:i32)  [unwired: 2 in, 2 out]
          n1334 = Less?(x=w403, y=317) -> (x < y?=w401:bool)
          n1335 = Or(x=w401, y=w400) -> (x .or. y?=w399:bool)
        }
        n1336 = local write "PESO\nNO"(FALSE ("PESO\nNO")) -> ()
        n1337 = local write "M53"(TRUE ("M53")) -> ()
        n1338 = local write "M52"(FALSE ("M52")) -> ()
      }
    }
    n1339 = case shown="True" w75 {
      frame False {
      }
      frame True {
        n1340 = while {
          stop <- w368 stop-if-true
          n1341 = property on="PINZA ABIERTA" class="Bool (strict)"() -> ("Left"=w391:i32)  [unwired: 2 in, 2 out]
          n1342 = Add(x=w391, y=9) -> (x+y=w389:i32)
          n1343 = property on="PINZA ABIERTA" class="Bool (strict)"("Left"=w389) -> ()  [unwired: 2 in, 2 out]
          n1344 = property on="VASTAGO RECHAZO" class="Bool (strict)"() -> ("Left"=w388:i32)  [unwired: 2 in, 2 out]
          n1345 = Add(x=w388, y=9) -> (x+y=w386:i32)
          n1346 = property on="VASTAGO RECHAZO" class="Bool (strict)"("Left"=w386) -> ()  [unwired: 2 in, 2 out]
          n1347 = property on="CILINDRO RECHAZO" class="Bool (strict)"() -> ("Left"=w385:i32)  [unwired: 2 in, 2 out]
          n1348 = Add(x=w385, y=9) -> (x+y=w383:i32)
          n1349 = property on="CILINDRO RECHAZO" class="Bool (strict)"("Left"=w383) -> ()  [unwired: 2 in, 2 out]
          n1350 = property on="CILINDRO RECHAZO1" class="Bool (strict)"() -> ("Left"=w382:i32)  [unwired: 2 in, 2 out]
          n1351 = Add(x=w382, y=9) -> (x+y=w380:i32)
          n1352 = property on="CILINDRO RECHAZO1" class="Bool (strict)"("Left"=w380) -> ()  [unwired: 2 in, 2 out]
          n1353 = property on="PINZA CERRADA" class="Bool (strict)"() -> ("Left"=w379:i32)  [unwired: 2 in, 2 out]
          n1354 = Add(x=w379, y=9) -> (x+y=w377:i32)
          n1355 = property on="PINZA CERRADA" class="Bool (strict)"("Left"=w377) -> ()  [unwired: 2 in, 2 out]
          n1356 = property on="ACTUADOR RECHAZO" class="Bool (strict)"() -> ("Top"=w376:i32)  [unwired: 2 in, 2 out]
          n1357 = Add(x=w376, y=9) -> (x+y=w374:i32)
          n1358 = property on="ACTUADOR RECHAZO" class="Bool (strict)"("Top"=w374) -> ()  [unwired: 2 in, 2 out]
          n1359 = Wait (ms)(milliseconds to wait=u32 0) -> ()  [unwired: 1 out]
          n1360 = local read "RESET"() -> (w369:bool)
          n1361 = property on="ACTUADOR RECHAZO" class="Bool (strict)"() -> ("Top"=w372:i32)  [unwired: 2 in, 2 out]
          n1362 = Greater?(x=w372, y=219) -> (0:w370:bool)
          n1363 = Or(x=w370, y=w369) -> (x .or. y?=w368:bool)
        }
        n1364 = local write "M53"(FALSE ("M53")) -> ()
        n1365 = local write "M54"(TRUE ("M54")) -> ()
      }
    }
    n1366 = property on="BNO COLOR" class="Bool (strict)"("Visible"=TRUE) -> ()  [unwired: 2 in, 2 out]
    n1367 = property on="BPESO SI" class="Bool (strict)"("Visible"=TRUE) -> ()  [unwired: 2 in, 2 out]
    n1368 = case shown="True" w313 {
      frame False {
      }
      frame True {
        n1369 = property on="estructura tapado" class="Bool (strict)"("Visible"=TRUE) -> ()  [unwired: 2 in, 2 out]
        n1370 = property on="tapa neutrop" class="Bool (strict)"("Visible"=TRUE) -> ()  [unwired: 2 in, 2 out]
        n1371 = property on="vastago1 tapado" class="Bool (strict)"("Visible"=TRUE) -> ()  [unwired: 2 in, 2 out]
        n1372 = property on="cilindro1 tapado" class="Bool (strict)"("Visible"=TRUE) -> ()  [unwired: 2 in, 2 out]
        n1373 = property on="vastago2 tapado" class="Bool (strict)"("Visible"=TRUE) -> ()  [unwired: 2 in, 2 out]
        n1374 = property on="cilindro2 tapado" class="Bool (strict)"("Visible"=TRUE) -> ()  [unwired: 2 in, 2 out]
        n1375 = property on="vastago3 tapado" class="Bool (strict)"("Visible"=TRUE) -> ()  [unwired: 2 in, 2 out]
        n1376 = property on="cilindro3 tapado" class="Bool (strict)"("Visible"=TRUE) -> ()  [unwired: 2 in, 2 out]
        n1377 = property on="vastago4 tapado" class="Bool (strict)"("Visible"=TRUE) -> ()  [unwired: 2 in, 2 out]
        n1378 = while {
          stop <- w1199 stop-if-true
          n1379 = property on="CILINDRO NUEVO" class="Bool (strict)"() -> ("Left"=w1222:i32)  [unwired: 2 in, 2 out]
          n1380 = Add(x=w1222, y=1) -> (x+y=w1200:i32)
          n1381 = property on="CILINDRO NUEVO" class="Bool (strict)"("Left"=w1200) -> ()  [unwired: 2 in, 2 out]
          n1382 = property on="BASTAGO TAPAS" class="Bool (strict)"() -> ("Left"=w1220:i32)  [unwired: 2 in, 2 out]
          n1383 = Subtract(x=w1220, y=3) -> (x-y=w1217:i32)
          n1384 = property on="BASTAGO TAPAS" class="Bool (strict)"("Left"=w1217) -> ()  [unwired: 2 in, 2 out]
          n1385 = property on="TAPA NEUTRO" class="Bool (strict)"() -> ("Left"=w1215:i32)  [unwired: 2 in, 2 out]
          n1386 = Subtract(x=w1215, y=3) -> (x-y=w1213:i32)
          n1387 = property on="TAPA NEUTRO" class="Bool (strict)"("Left"=w1213) -> ()  [unwired: 2 in, 2 out]
          n1388 = property on="vastago1 tapado" class="Bool (strict)"() -> ("Left"=w1210:i32)  [unwired: 2 in, 2 out]
          n1389 = Add(x=w1210, y=3) -> (x+y=w1208:i32)
          n1390 = property on="vastago1 tapado" class="Bool (strict)"("Left"=w1208) -> ()  [unwired: 2 in, 2 out]
          n1391 = property on="tapa neutrop" class="Bool (strict)"() -> ("Left"=w1207:i32)  [unwired: 2 in, 2 out]
          n1392 = Add(x=w1207, y=3) -> (x+y=w1205:i32)
          n1393 = property on="tapa neutrop" class="Bool (strict)"("Left"=w1205) -> ()  [unwired: 2 in, 2 out]
          n1394 = property on="vastago2 tapado" class="Bool (strict)"() -> ("Left"=w1204:i32)  [unwired: 2 in, 2 out]
          n1395 = Subtract(x=w1204, y=1) -> (x-y=w1202:i32)
          n1396 = property on="vastago2 tapado" class="Bool (strict)"("Left"=w1202) -> ()  [unwired: 2 in, 2 out]
          n1397 = Wait (ms)(milliseconds to wait=u32 0) -> ()  [unwired: 1 out]
          n1398 = local read "RESET"() -> (w1211:bool)
          n1399 = property on="BASTAGO TAPAS" class="Bool (strict)"() -> ("Left"=w1216:i32)  [unwired: 2 in, 2 out]
          n1400 = Less?(x=w1216, y=911) -> (x < y?=w1212:bool)
          n1401 = Or(x=w1212, y=w1211) -> (x .or. y?=w1199:bool)
        }
        n1402 = local write "M9"(FALSE ("M9")) -> ()
        n1403 = local write "M10"(TRUE ("M10")) -> ()
      }
    }
    n1404 = case shown="True" w162 {
      frame False {
      }
      frame True {
        n1405 = property on="CILINDRO RECHAZO1" class="Bool (strict)"("Visible"=TRUE) -> ()  [unwired: 2 in, 2 out]
        n1406 = property on="ESTRUCTURA RECHAZO" class="Bool (strict)"("Visible"=TRUE) -> ()  [unwired: 2 in, 2 out]
        n1407 = property on="CILINDRO RECHAZO" class="Bool (strict)"("Visible"=TRUE) -> ()  [unwired: 2 in, 2 out]
        n1408 = property on="TARRO NOCOLOR" class="Bool (strict)"("Visible"=TRUE) -> ()  [unwired: 2 in, 2 out]
        n1409 = property on="PINZA ABIERTA" class="Bool (strict)"("Visible"=TRUE) -> ()  [unwired: 2 in, 2 out]
        n1410 = property on="VASTAGO RECHAZO" class="Bool (strict)"("Visible"=TRUE) -> ()  [unwired: 2 in, 2 out]
        n1411 = property on="DEPOSITO NOCOLOR" class="Bool (strict)"("Visible"=TRUE) -> ()  [unwired: 2 in, 2 out]
        n1412 = property on="DEPOSITO NOPESO" class="Bool (strict)"("Visible"=TRUE) -> ()  [unwired: 2 in, 2 out]
        n1413 = while {
          stop <- w739 stop-if-true
          n1414 = property on="CILINDRO RECHAZO1" class="Bool (strict)"() -> ("Left"=w762:i32)  [unwired: 2 in, 2 out]
          n1415 = Subtract(x=w762, y=9) -> (x-y=w760:i32)
          n1416 = property on="CILINDRO RECHAZO1" class="Bool (strict)"("Left"=w760) -> ()  [unwired: 2 in, 2 out]
          n1417 = property on="PINZA CERRADA" class="Bool (strict)"() -> ("Left"=w759:i32)  [unwired: 2 in, 2 out]
          n1418 = Subtract(x=w759, y=9) -> (x-y=w757:i32)
          n1419 = property on="PINZA CERRADA" class="Bool (strict)"("Left"=w757) -> ()  [unwired: 2 in, 2 out]
          n1420 = property on="CILINDRO RECHAZO" class="Bool (strict)"() -> ("Left"=w756:i32)  [unwired: 2 in, 2 out]
          n1421 = Subtract(x=w756, y=9) -> (x-y=w754:i32)
          n1422 = property on="CILINDRO RECHAZO" class="Bool (strict)"("Left"=w754) -> ()  [unwired: 2 in, 2 out]
          n1423 = property on="VASTAGO RECHAZO" class="Bool (strict)"() -> ("Left"=w753:i32)  [unwired: 2 in, 2 out]
          n1424 = Subtract(x=w753, y=9) -> (x-y=w751:i32)
          n1425 = property on="VASTAGO RECHAZO" class="Bool (strict)"("Left"=w751) -> ()  [unwired: 2 in, 2 out]
          n1426 = property on="PINZA ABIERTA" class="Bool (strict)"() -> ("Left"=w750:i32)  [unwired: 2 in, 2 out]
          n1427 = Subtract(x=w750, y=9) -> (x-y=w748:i32)
          n1428 = property on="PINZA ABIERTA" class="Bool (strict)"("Left"=w748) -> ()  [unwired: 2 in, 2 out]
          n1429 = property on="ACTUADOR RECHAZO" class="Bool (strict)"() -> ("Top"=w747:i32)  [unwired: 2 in, 2 out]
          n1430 = Subtract(x=w747, y=9) -> (x-y=w745:i32)
          n1431 = property on="ACTUADOR RECHAZO" class="Bool (strict)"("Top"=w745) -> ()  [unwired: 2 in, 2 out]
          n1432 = Wait (ms)(milliseconds to wait=u32 0) -> ()  [unwired: 1 out]
          n1433 = local read "RESET"() -> (w740:bool)
          n1434 = property on="ACTUADOR RECHAZO" class="Bool (strict)"() -> ("Top"=w743:i32)  [unwired: 2 in, 2 out]
          n1435 = Less?(x=w743, y=6) -> (x < y?=w741:bool)
          n1436 = Or(x=w741, y=w740) -> (x .or. y?=w739:bool)
        }
        n1437 = local write "M37"(FALSE ("M37")) -> ()
        n1438 = local write "M38"(TRUE ("M38")) -> ()
      }
    }
    n1439 = case shown="True" w147 {
      frame False {
      }
      frame True {
        n1440 = while {
          stop <- w661 stop-if-true
          n1441 = property on="PINZA ABIERTA" class="Bool (strict)"() -> ("Left"=w690:i32)  [unwired: 2 in, 2 out]
          n1442 = Add(x=w690, y=12) -> (x+y=w688:i32)
          n1443 = property on="PINZA ABIERTA" class="Bool (strict)"("Left"=w688) -> ()  [unwired: 2 in, 2 out]
          n1444 = property on="VASTAGO RECHAZO" class="Bool (strict)"() -> ("Left"=w687:i32)  [unwired: 2 in, 2 out]
          n1445 = Add(x=w687, y=12) -> (x+y=w685:i32)
          n1446 = property on="VASTAGO RECHAZO" class="Bool (strict)"("Left"=w685) -> ()  [unwired: 2 in, 2 out]
          n1447 = property on="TARRO NOCOLOR" class="Bool (strict)"() -> ("Left"=w684:i32)  [unwired: 2 in, 2 out]
          n1448 = Add(x=w684, y=12) -> (x+y=w682:i32)
          n1449 = property on="TARRO NOCOLOR" class="Bool (strict)"("Left"=w682) -> ()  [unwired: 2 in, 2 out]
          n1450 = property on="TAPA NOCOLOR" class="Bool (strict)"() -> ("Top"=w681:i32)  [unwired: 2 in, 2 out]
          n1451 = Add(x=w681, y=12) -> (x+y=w679:i32)
          n1452 = property on="TAPA NOCOLOR" class="Bool (strict)"("Top"=w679) -> ()  [unwired: 2 in, 2 out]
          n1453 = property on="CILINDRO RECHAZO" class="Bool (strict)"() -> ("Left"=w678:i32)  [unwired: 2 in, 2 out]
          n1454 = Add(x=w678, y=12) -> (x+y=w676:i32)
          n1455 = property on="CILINDRO RECHAZO" class="Bool (strict)"("Left"=w676) -> ()  [unwired: 2 in, 2 out]
          n1456 = property on="PINZA CERRADA" class="Bool (strict)"() -> ("Left"=w675:i32)  [unwired: 2 in, 2 out]
          n1457 = Add(x=w675, y=12) -> (x+y=w673:i32)
          n1458 = property on="PINZA CERRADA" class="Bool (strict)"("Left"=w673) -> ()  [unwired: 2 in, 2 out]
          n1459 = property on="CILINDRO RECHAZO1" class="Bool (strict)"() -> ("Left"=w672:i32)  [unwired: 2 in, 2 out]
          n1460 = Add(x=w672, y=12) -> (x+y=w670:i32)
          n1461 = property on="CILINDRO RECHAZO1" class="Bool (strict)"("Left"=w670) -> ()  [unwired: 2 in, 2 out]
          n1462 = property on="ACTUADOR RECHAZO" class="Bool (strict)"() -> ("Top"=w669:i32)  [unwired: 2 in, 2 out]
          n1463 = Add(x=w669, y=12) -> (x+y=w667:i32)
          n1464 = property on="ACTUADOR RECHAZO" class="Bool (strict)"("Top"=w667) -> ()  [unwired: 2 in, 2 out]
          n1465 = Wait (ms)(milliseconds to wait=u32 0) -> ()  [unwired: 1 out]
          n1466 = local read "RESET"() -> (w662:bool)
          n1467 = property on="ACTUADOR RECHAZO" class="Bool (strict)"() -> ("Top"=w665:i32)  [unwired: 2 in, 2 out]
          n1468 = Greater?(x=w665, y=219) -> (0:w663:bool)
          n1469 = Or(x=w663, y=w662) -> (x .or. y?=w661:bool)
        }
        n1470 = local write "M40"(FALSE ("M40")) -> ()
        n1471 = local write "M41"(TRUE ("M41")) -> ()
      }
    }
    n1472 = case shown="True" w105 {
      frame False {
      }
      frame True {
        n1473 = property on="CILINDRO RECHAZO1" class="Bool (strict)"("Visible"=TRUE) -> ()  [unwired: 2 in, 2 out]
        n1474 = property on="ESTRUCTURA RECHAZO" class="Bool (strict)"("Visible"=TRUE) -> ()  [unwired: 2 in, 2 out]
        n1475 = property on="CILINDRO RECHAZO" class="Bool (strict)"("Visible"=TRUE) -> ()  [unwired: 2 in, 2 out]
        n1476 = property on="TARRO NOPESO" class="Bool (strict)"("Visible"=TRUE) -> ()  [unwired: 2 in, 2 out]
        n1477 = property on="PINZA ABIERTA" class="Bool (strict)"("Visible"=TRUE) -> ()  [unwired: 2 in, 2 out]
        n1478 = property on="VASTAGO RECHAZO" class="Bool (strict)"("Visible"=TRUE) -> ()  [unwired: 2 in, 2 out]
        n1479 = property on="DEPOSITO NOCOLOR" class="Bool (strict)"("Visible"=TRUE) -> ()  [unwired: 2 in, 2 out]
        n1480 = property on="DEPOSITO NOPESO" class="Bool (strict)"("Visible"=TRUE) -> ()  [unwired: 2 in, 2 out]
        n1481 = while {
          stop <- w518 stop-if-true
          n1482 = property on="CILINDRO RECHAZO1" class="Bool (strict)"() -> ("Left"=w538:i32)  [unwired: 2 in, 2 out]
          n1483 = Subtract(x=w538, y=9) -> (x-y=w536:i32)
          n1484 = property on="CILINDRO RECHAZO1" class="Bool (strict)"("Left"=w536) -> ()  [unwired: 2 in, 2 out]
          n1485 = property on="PINZA CERRADA" class="Bool (strict)"() -> ("Left"=w535:i32)  [unwired: 2 in, 2 out]
          n1486 = Subtract(x=w535, y=9) -> (x-y=w533:i32)
          n1487 = property on="PINZA CERRADA" class="Bool (strict)"("Left"=w533) -> ()  [unwired: 2 in, 2 out]
          n1488 = property on="CILINDRO RECHAZO" class="Bool (strict)"() -> ("Left"=w532:i32)  [unwired: 2 in, 2 out]
          n1489 = Subtract(x=w532, y=9) -> (x-y=w530:i32)
          n1490 = property on="CILINDRO RECHAZO" class="Bool (strict)"("Left"=w530) -> ()  [unwired: 2 in, 2 out]
          n1491 = property on="VASTAGO RECHAZO" class="Bool (strict)"() -> ("Left"=w529:i32)  [unwired: 2 in, 2 out]
          n1492 = Subtract(x=w529, y=9) -> (x-y=w527:i32)
          n1493 = property on="VASTAGO RECHAZO" class="Bool (strict)"("Left"=w527) -> ()  [unwired: 2 in, 2 out]
          n1494 = property on="PINZA ABIERTA" class="Bool (strict)"() -> ("Left"=w526:i32)  [unwired: 2 in, 2 out]
          n1495 = Subtract(x=w526, y=9) -> (x-y=w524:i32)
          n1496 = property on="PINZA ABIERTA" class="Bool (strict)"("Left"=w524) -> ()  [unwired: 2 in, 2 out]
          n1497 = property on="ACTUADOR RECHAZO" class="Bool (strict)"() -> ("Top"=w517:i32)  [unwired: 2 in, 2 out]
          n1498 = Subtract(x=w517, y=9) -> (x-y=w516:i32)
          n1499 = property on="ACTUADOR RECHAZO" class="Bool (strict)"("Top"=w516) -> ()  [unwired: 2 in, 2 out]
          n1500 = Wait (ms)(milliseconds to wait=u32 0) -> ()  [unwired: 1 out]
          n1501 = local read "RESET"() -> (w519:bool)
          n1502 = property on="ACTUADOR RECHAZO" class="Bool (strict)"() -> ("Top"=w515:i32)  [unwired: 2 in, 2 out]
          n1503 = Less?(x=w515, y=6) -> (x < y?=w520:bool)
          n1504 = Or(x=w520, y=w519) -> (x .or. y?=w518:bool)
        }
        n1505 = local write "M47"(FALSE ("M47")) -> ()
        n1506 = local write "M48"(TRUE ("M48")) -> ()
      }
    }
    n1507 = case shown="True" w90 {
      frame False {
      }
      frame True {
        n1508 = while {
          stop <- w438 stop-if-true
          n1509 = property on="PINZA ABIERTA" class="Bool (strict)"() -> ("Left"=w465:i32)  [unwired: 2 in, 2 out]
          n1510 = Add(x=w465, y=9) -> (x+y=w463:i32)
          n1511 = property on="PINZA ABIERTA" class="Bool (strict)"("Left"=w463) -> ()  [unwired: 2 in, 2 out]
          n1512 = property on="VASTAGO RECHAZO" class="Bool (strict)"() -> ("Left"=w462:i32)  [unwired: 2 in, 2 out]
          n1513 = Add(x=w462, y=9) -> (x+y=w460:i32)
          n1514 = property on="VASTAGO RECHAZO" class="Bool (strict)"("Left"=w460) -> ()  [unwired: 2 in, 2 out]
          n1515 = property on="TARRO NOPESO" class="Bool (strict)"() -> ("Left"=w459:i32)  [unwired: 2 in, 2 out]
          n1516 = Add(x=w459, y=9) -> (x+y=w457:i32)
          n1517 = property on="TARRO NOPESO" class="Bool (strict)"("Left"=w457) -> ()  [unwired: 2 in, 2 out]
          n1518 = property on="TAPA NOPESO" class="Bool (strict)"() -> ("Top"=w437:i32)  [unwired: 2 in, 2 out]
          n1519 = Add(x=w437, y=9) -> (x+y=w436:i32)
          n1520 = property on="TAPA NOPESO" class="Bool (strict)"("Top"=w436) -> ()  [unwired: 2 in, 2 out]
          n1521 = property on="CILINDRO RECHAZO" class="Bool (strict)"() -> ("Left"=w455:i32)  [unwired: 2 in, 2 out]
          n1522 = Add(x=w455, y=9) -> (x+y=w453:i32)
          n1523 = property on="CILINDRO RECHAZO" class="Bool (strict)"("Left"=w453) -> ()  [unwired: 2 in, 2 out]
          n1524 = property on="PINZA CERRADA" class="Bool (strict)"() -> ("Left"=w452:i32)  [unwired: 2 in, 2 out]
          n1525 = Add(x=w452, y=9) -> (x+y=w450:i32)
          n1526 = property on="PINZA CERRADA" class="Bool (strict)"("Left"=w450) -> ()  [unwired: 2 in, 2 out]
          n1527 = property on="CILINDRO RECHAZO1" class="Bool (strict)"() -> ("Left"=w449:i32)  [unwired: 2 in, 2 out]
          n1528 = Add(x=w449, y=9) -> (x+y=w447:i32)
          n1529 = property on="CILINDRO RECHAZO1" class="Bool (strict)"("Left"=w447) -> ()  [unwired: 2 in, 2 out]
          n1530 = property on="ACTUADOR RECHAZO" class="Bool (strict)"() -> ("Top"=w446:i32)  [unwired: 2 in, 2 out]
          n1531 = Add(x=w446, y=9) -> (x+y=w444:i32)
          n1532 = property on="ACTUADOR RECHAZO" class="Bool (strict)"("Top"=w444) -> ()  [unwired: 2 in, 2 out]
          n1533 = Wait (ms)(milliseconds to wait=u32 0) -> ()  [unwired: 1 out]
          n1534 = local read "RESET"() -> (w439:bool)
          n1535 = property on="ACTUADOR RECHAZO" class="Bool (strict)"() -> ("Top"=w442:i32)  [unwired: 2 in, 2 out]
          n1536 = Greater?(x=w442, y=100) -> (0:w440:bool)
          n1537 = Or(x=w440, y=w439) -> (x .or. y?=w438:bool)
        }
        n1538 = local write "M50"(FALSE ("M50")) -> ()
        n1539 = local write "M51"(TRUE ("M51")) -> ()
      }
    }
    n1540 = property on="BPESO NO" class="Bool (strict)"("Visible"=TRUE) -> ()  [unwired: 2 in, 2 out]
    n1541 = local read "REINICIAR\nCONTEO"() -> (w354:bool)
    n1542 = case shown="True" w354 {
      frame False {
      }
      frame True {
        n1543 = local read "FINALIZADOS\nAZULES"() -> (w1536:dbl)
        n1544 = local read "FINALIZADOS\nROJOS"() -> (w1538:dbl)
        n1545 = local read "FINALIZADOS\nRECHAZADOS"() -> (w1540:dbl)
        n1546 = Multiply(x=w1536, y=0.0) -> (x*y=w1534:dbl)
        n1547 = Multiply(x=w1538, y=0.0) -> (x*y=w1533:dbl)
        n1548 = Multiply(x=w1540, y=0.0) -> (x*y=w1532:dbl)
        n1549 = local write "FINALIZADOS\nAZULES"(w1534) -> ()
        n1550 = local write "FINALIZADOS\nROJOS"(w1533) -> ()
        n1551 = local write "FINALIZADOS\nRECHAZADOS"(w1532) -> ()
      }
    }
  }
